vi "指令集合.vi"() -> ()   [LabVIEW 2016]
uses:
  Global variable.vi
  <vilib>/addons/_office/excel.llb/Excel Get Data ([str]).vi
  <vilib>/regexp/Match Regular Expression.xnode
  <vilib>/Utility/NIReport.llb/NI_report.lvclass
  <vilib>/Utility/NIReport.llb/Excel/NI_Excel.lvclass
  <vilib>/addons/_office/NI_ReportGenerationToolkit.lvlib
panel:
  in  "Tab Control":T1(tab)
  in  "get_error":bool
  in  "ooc or b update":enum16{"b update", "ooc update", "ooc&b update"}(ring)
  in  "打快门":bool
  in  "数据源":T2(ring)
  in  "byPathSel":enum16{"0", "1"}(ring)=enum."1"
  in  "KBC":bool=TRUE
  in  "AGC":bool=TRUE
  in  "HBC":bool=TRUE
  in  "VBC":bool=TRUE
  in  "TNR":bool=TRUE
  in  "SNR":bool=TRUE
  in  "GAMMA":bool=TRUE
  in  "像素取反":bool
  in  "去锅盖":bool=TRUE
  in  "对焦使能":bool
  in  "Blind_rp_en":bool
  in  "VISA resource name":refnum<visa-resource-name>
  in  "COM":bool
  in  "快门片使能":bool=TRUE
  in  "快门片开合":bool=TRUE
  in  "get_vtemp":bool
  out "return":i32
  out "vtemp":u16
  in  "命令集合":string(combo)
  in  "指令窗口":string
  out "指令触发":bool
  out "error out":errorcluster
  in  "new_dead_pix":u8[](array[numeric])
  out "String_out":string
  in  "String_in":string
  in  "Enum":enum16{"number", "hex", "string"}(ring)
  in  "数值":u8
  in  "长度":u16
  in  "加载到data_in":bool
  in  "data数组清空":bool
  out "data_out":u8[](array[numeric])
  in  "data_in":u8[](array[numeric])
  in  "standard_get":bool
  in  "standard_send":bool
  in  "std_byCmdType":string
  in  "std_bySubCmd":string
  in  "std_byPara":string
  in  "std_byAddr_h":string
  in  "std_wAddr":string
  in  "std_wLength":string
  in  "cmd_std_header_t":T3
  out "standard_send_return":i32
  out "standard_get_return":i32
  in  "Boolean":bool
  out "读取字符串（16进制）":string
  in  "写入字符串（16进制）":string
  in  "写入长度":string
  in  "写入地址（16进制）":string
  in  "读取地址（16进制）":string
  in  "读取长度":string
  in  "寄存器写入":bool
  in  "寄存器读取":bool
  in  "long_dwLen":string
  in  "long_dwAddr2":string
  in  "long_dwAddr1":string
  in  "long_wPara":string
  in  "long_bySubCmd":string
  in  "long_byCmd":string
  in  "long_get":bool
  in  "long_send":bool
  in  "vd_cmd_long_header_t":T4
  out "long_send_return":i32
  out "long_data out":u8[](array[numeric])
  out "long_get_return":i32
  in  "osd_get":bool
  in  "osd_send":bool
  out "osd_get_return":i32
  out "osd_data out":u8[](array[numeric])
  out "osd_send_return":i32
  in  "osd_byCmd":string
  in  "osd_bySubcmd":string
  in  "osd_byIndex":string
  in  "osd_byPara":string
  in  "osd_data_in":u8[](array[numeric])
  out "快门开合":i32
  out "快门使能":i32
  out "Blind_rp_en R":i32
  out "像素取反 return":i32
  out "读取寄存器":i32
  out "写入寄存器":i32
  out "GAMMA return":i32
  out "AGC return":i32
  out "SNR return":i32
  out "TNR return":i32
  out "VBC return":i32
  out "HBC return":i32
  out "去锅盖 return":i32
  out "KBC return":i32
  out "对焦使能 2":i32
  out "Y16start":i32
  out "Y16stop":i32
  out "oocBupdate":i32
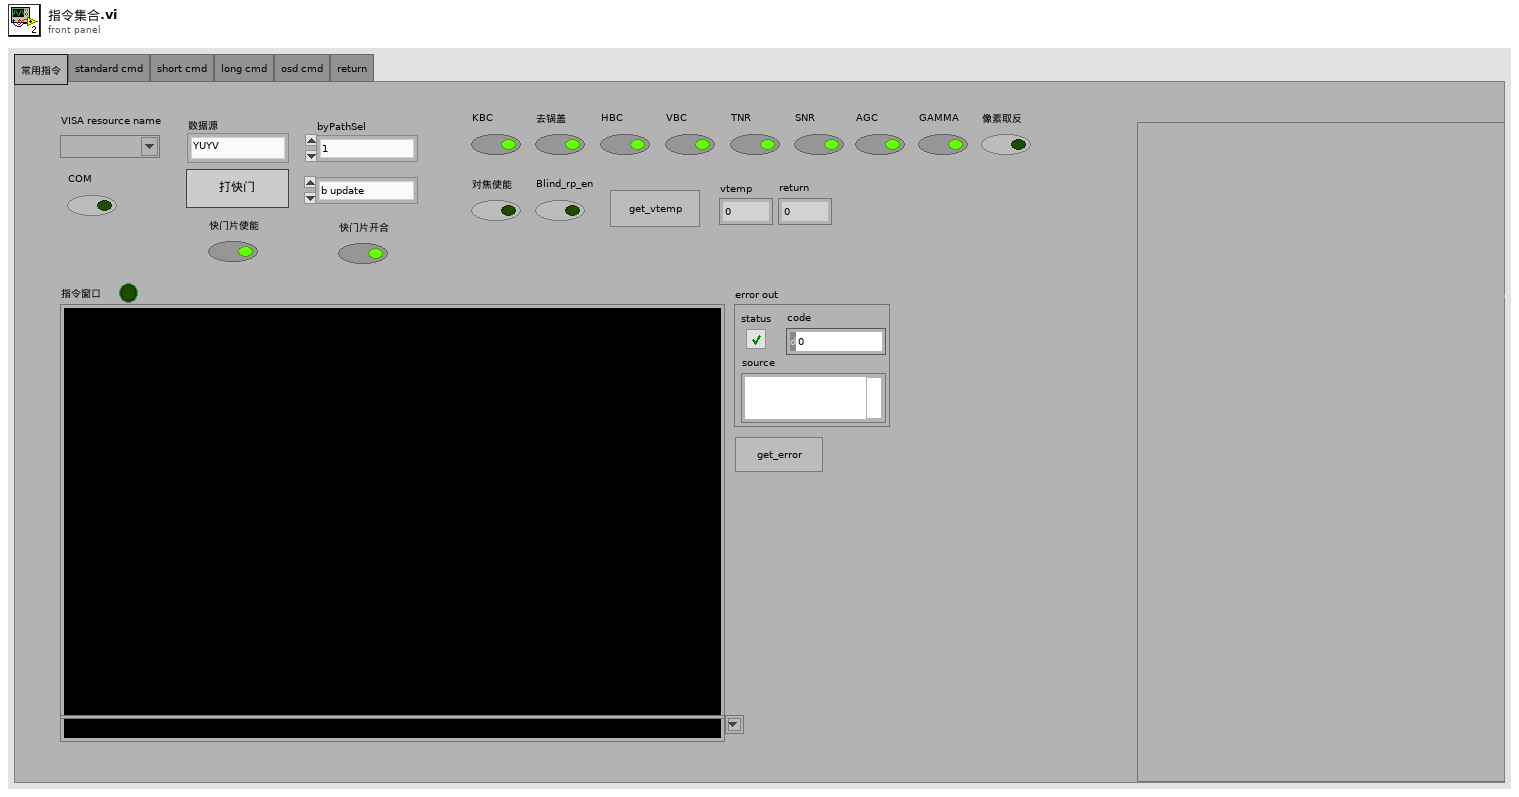
[diagram p1: front panel]
types:
  T1 = enum32{"常用指令", "standard cmd", "short cmd", "long cmd", "osd cmd", "return"}
  T2 = enum16{"YUYV", "TEMPERATURE", "IR", "KBC", "HBC_DPC", "VBC", "TNR", "SNR", "AGC", "DDE", "GAMMA", "MIRROR"}
  T3 = cluster{"byCmdType":u8, "bySubCmd":u8, "byPara":u8, "byAddr_h":u8, "byAddr_l":u8, "byAddr_ll":u8, "byLen_h":u8, "byLen_l":u8}
  T4 = cluster{"byCmd":u8, "bySubCmd":u8, "byParam_h":u8, "byParam_l":u8, "byAddr1_hh":u8, "byAddr1_h":u8, "byAddr1_l":u8, "byAddr1_ll":u8, "byAddr2_hh":u8, "byAddr2_h":u8, "byAddr2_l":u8, "byAddr2_ll":u8, "byLen_hh":u8, "byLen_h":u8, "byLen_l":u8, "byLen_ll":u8}
  T5 = enum16{"Standard Report", "HTML", "Word", "Excel"}
  T6 = enum16{"maximized", "minimized", "normal", "no change"}
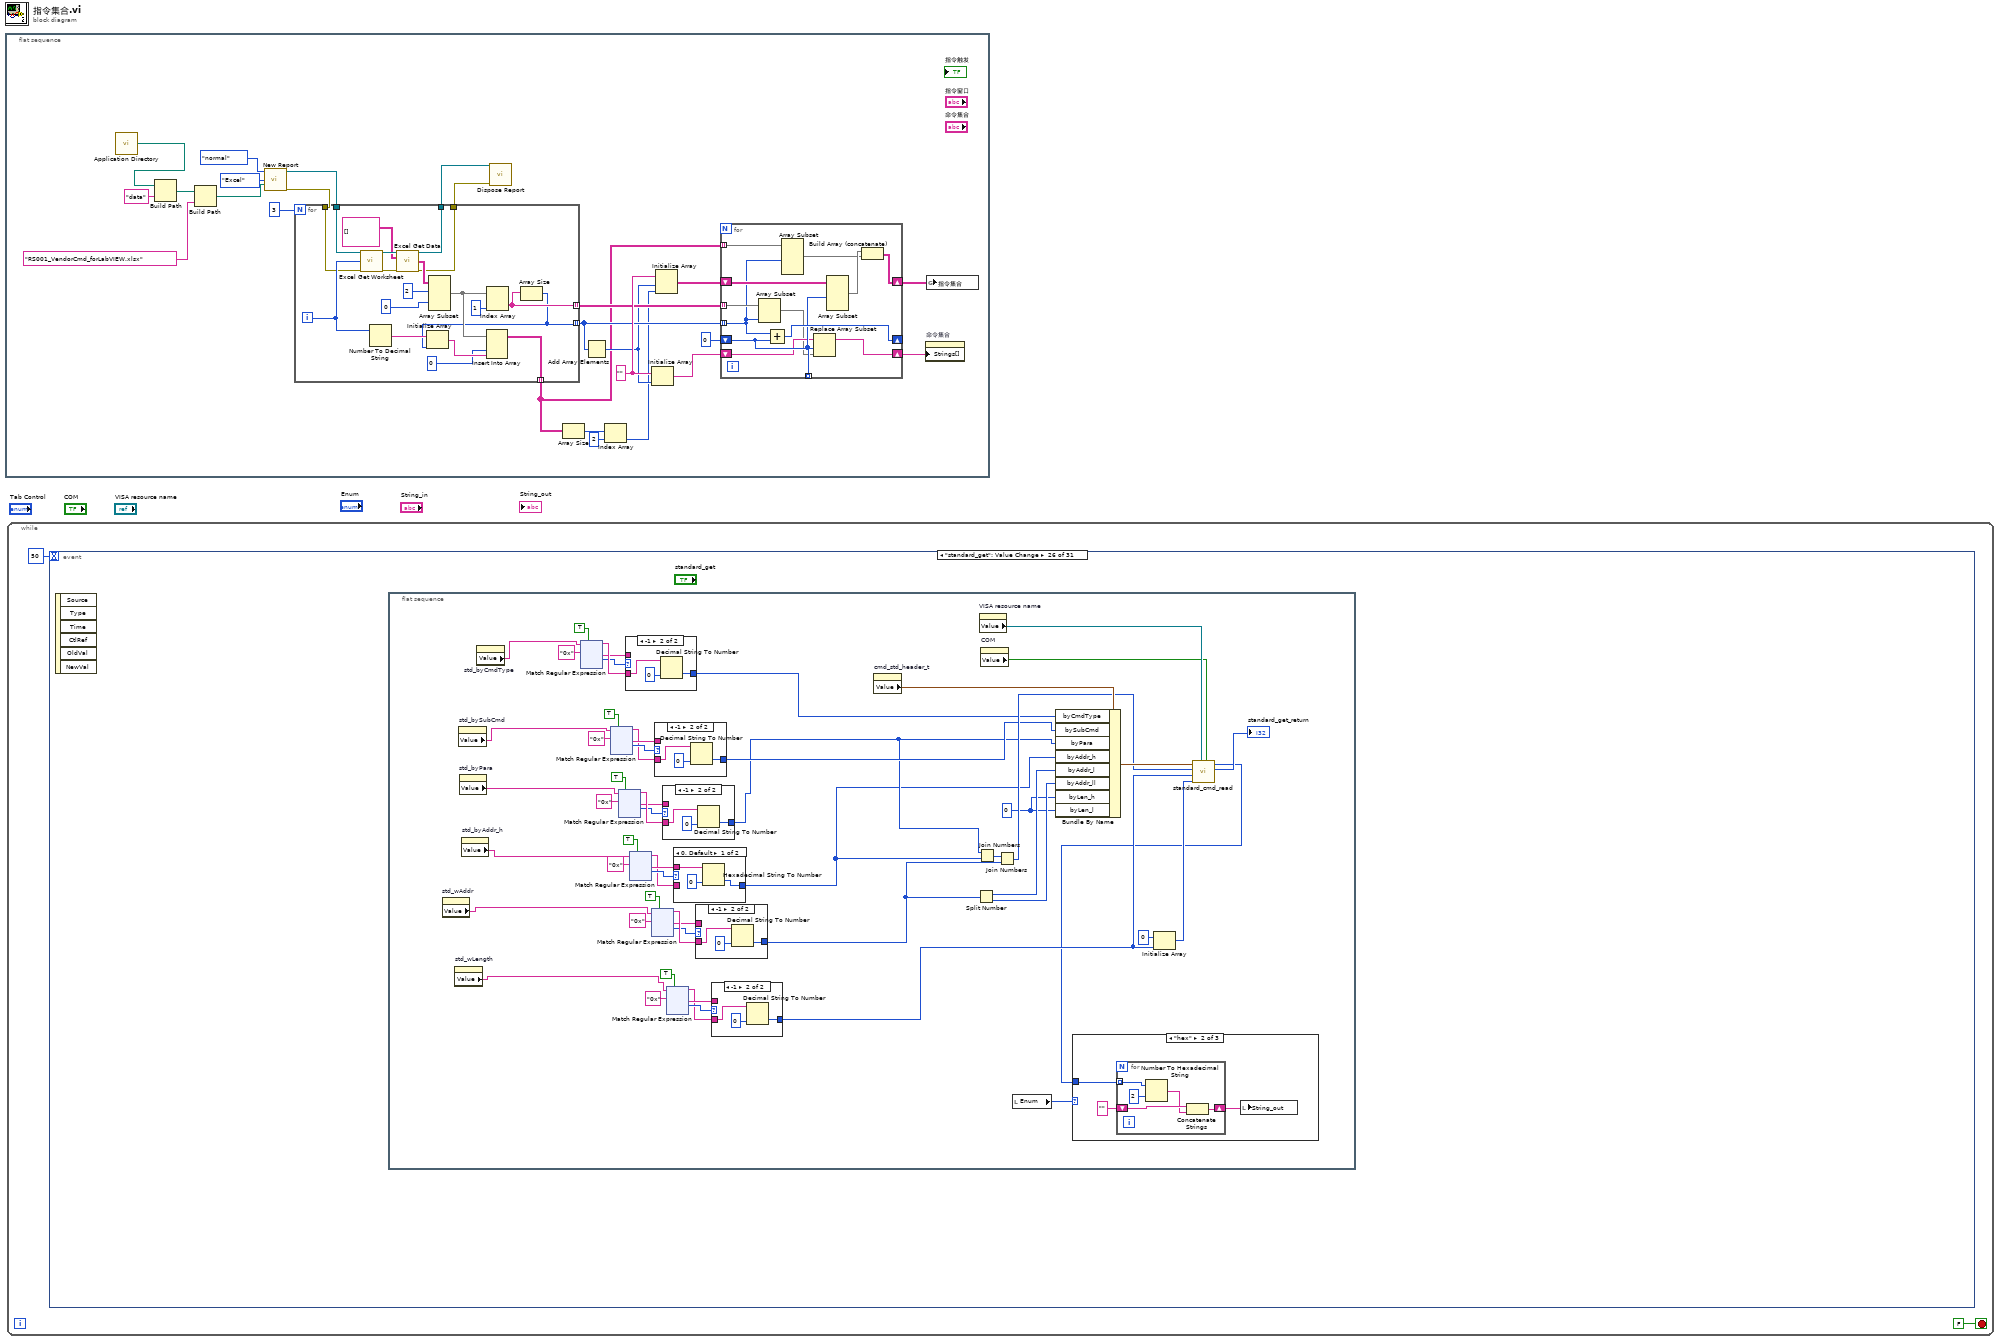
[diagram p0: block diagram]
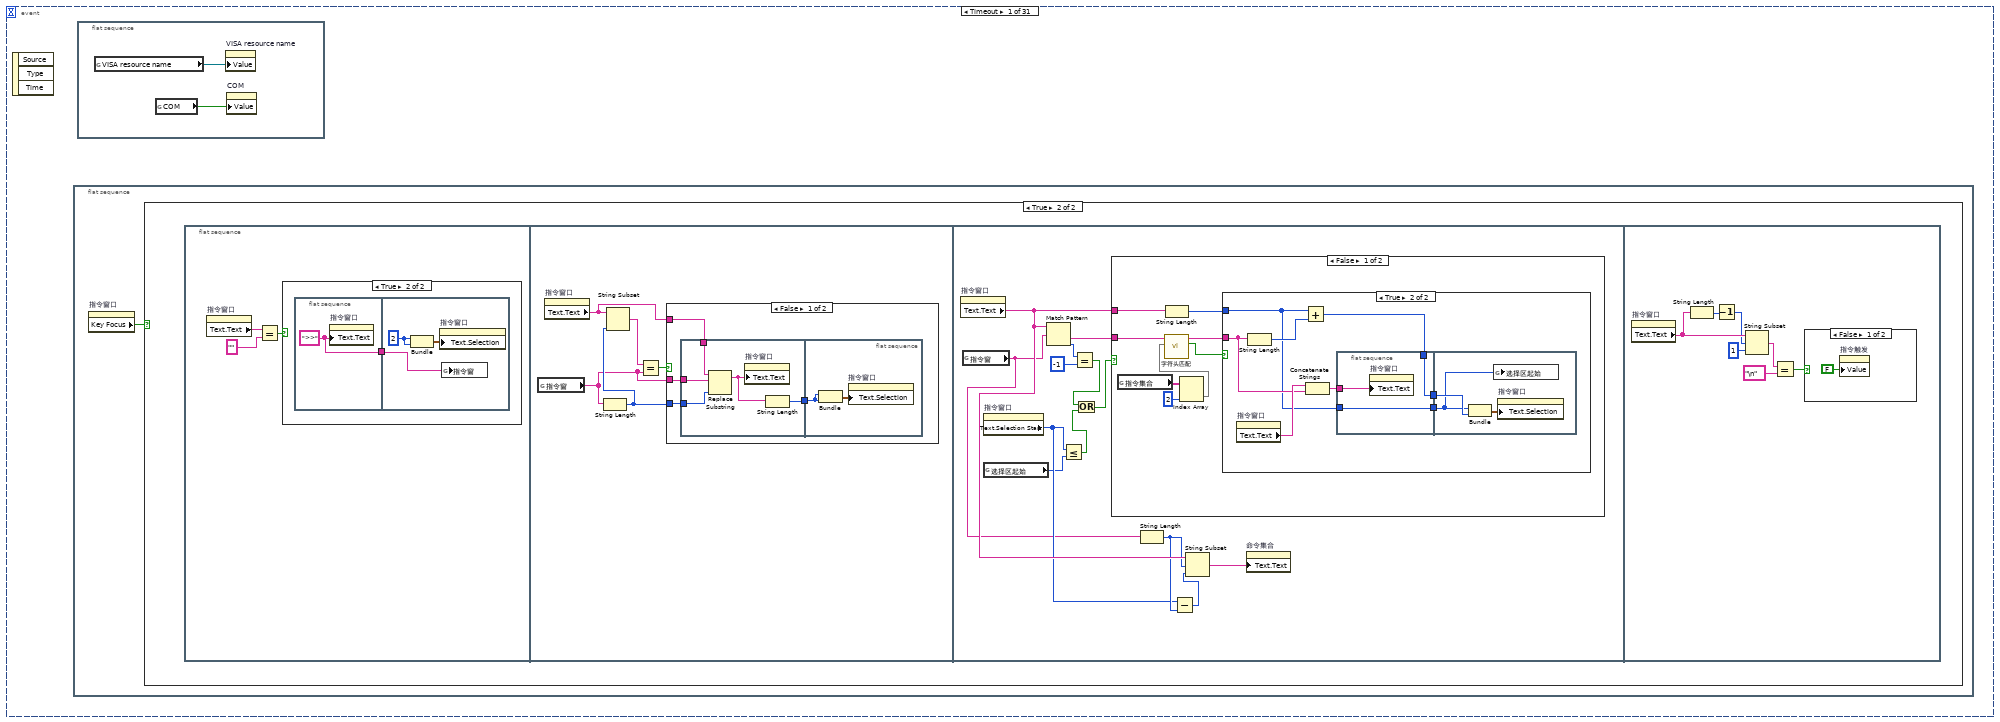
[diagram p2: hidden frame]
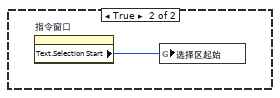
[diagram p7: hidden frame]
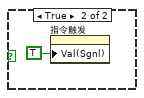
[diagram p8: hidden frame]
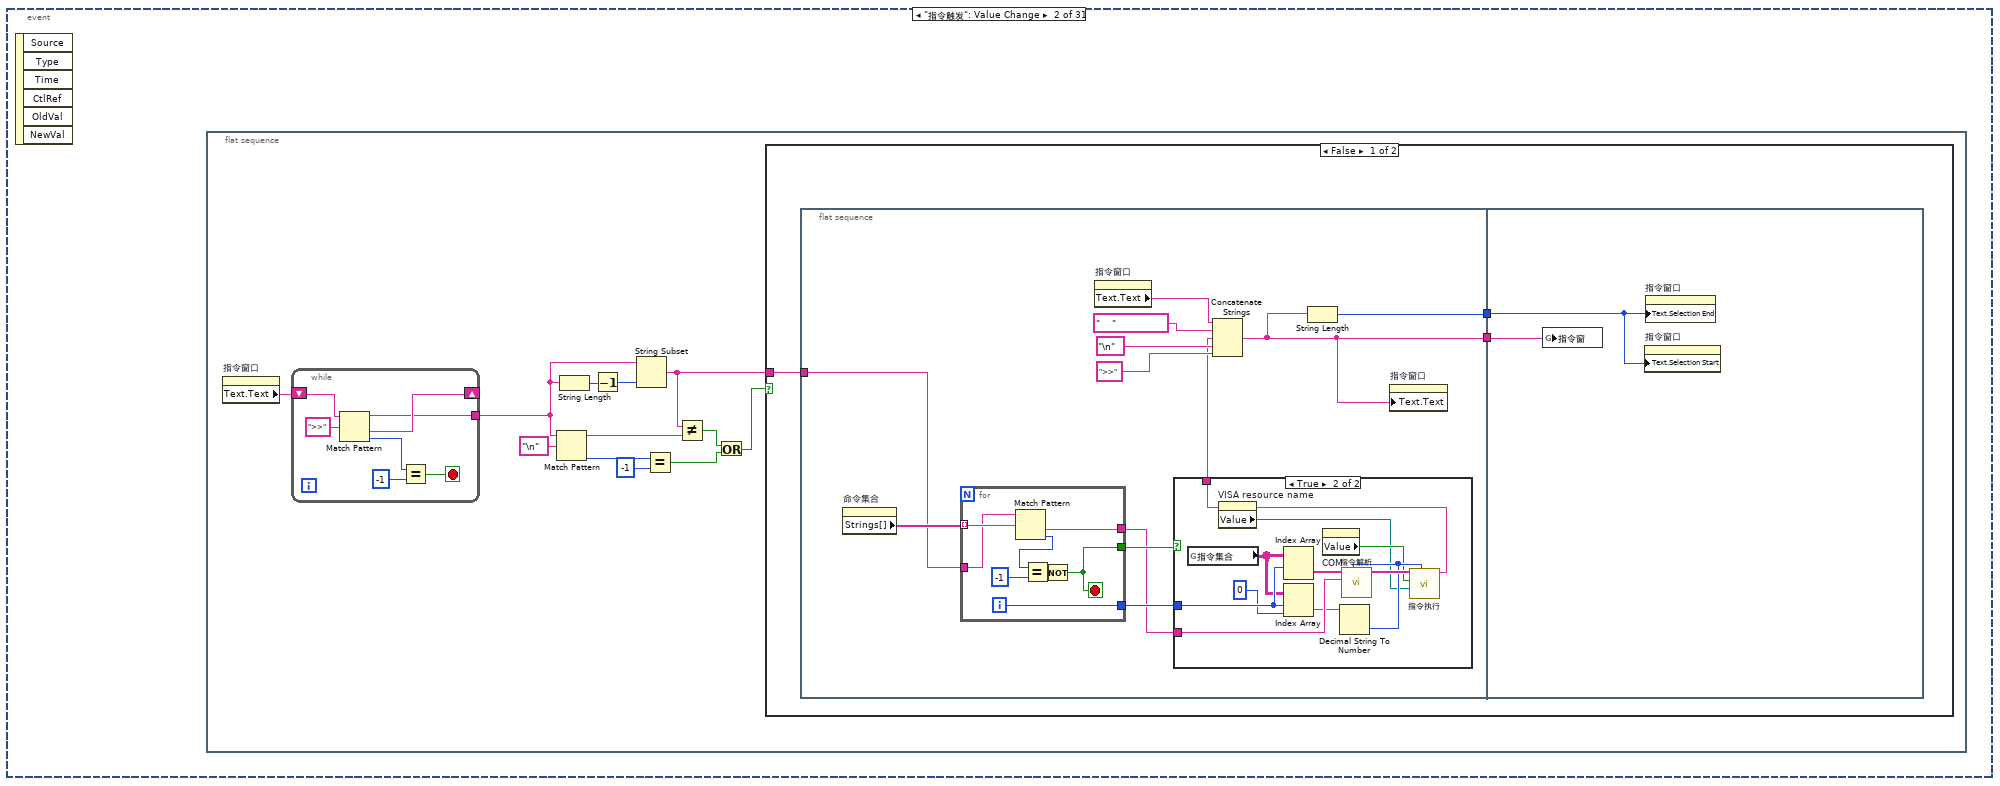
[diagram p9: hidden frame]
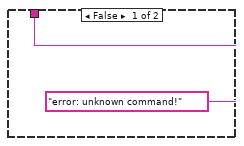
[diagram p10: hidden frame]
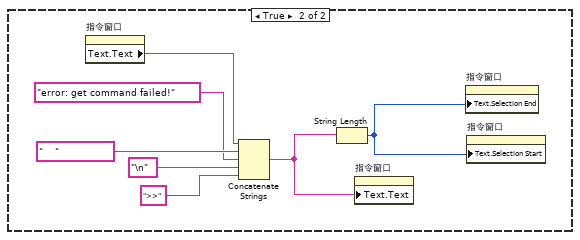
[diagram p11: hidden frame]
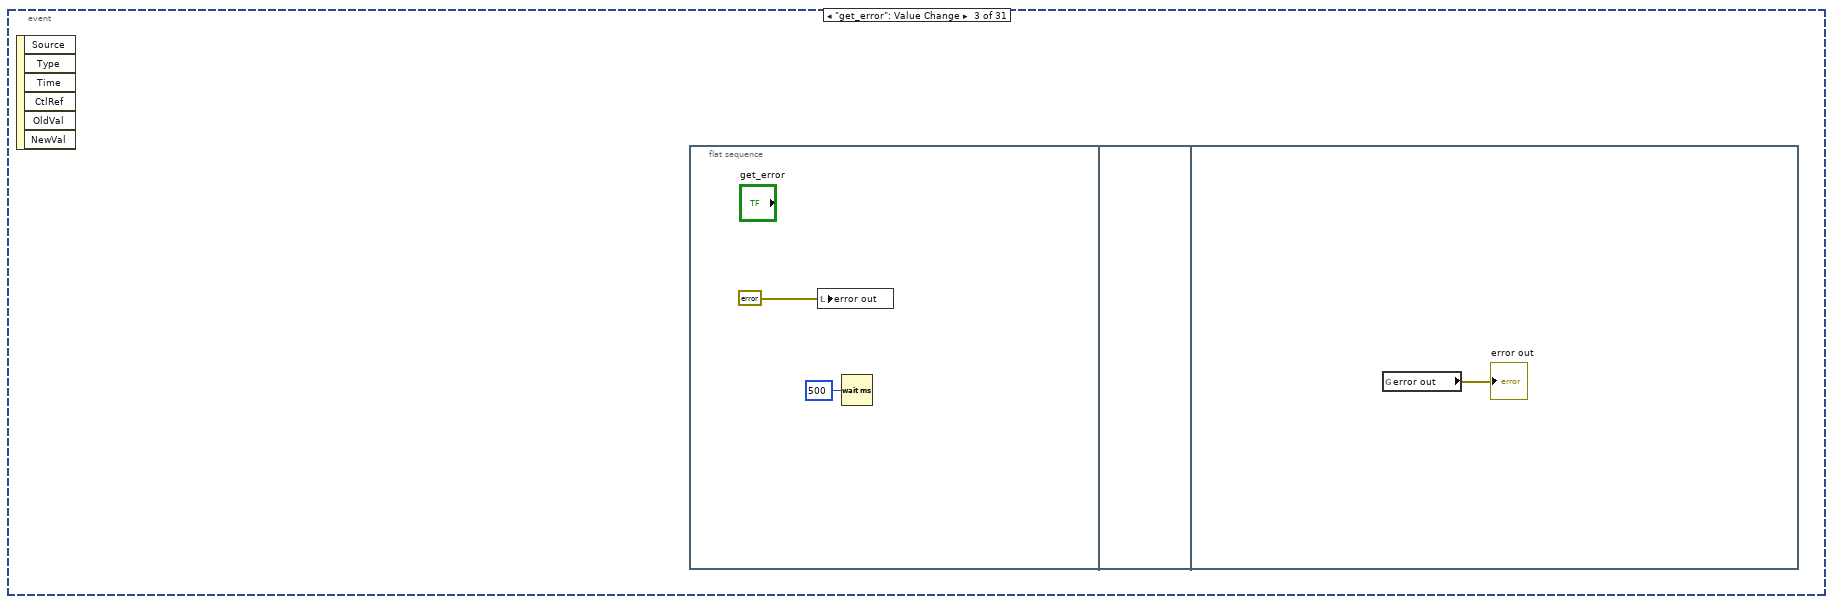
[diagram p12: hidden frame]
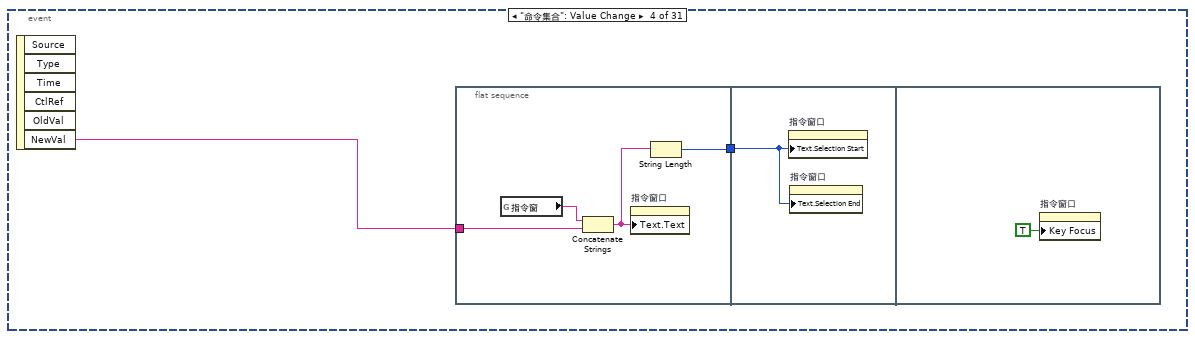
[diagram p13: hidden frame]
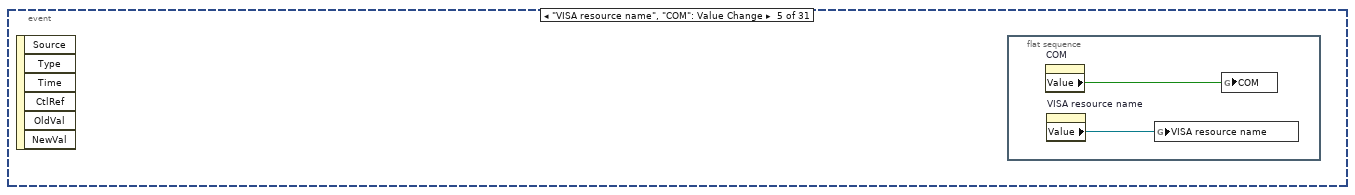
[diagram p14: hidden frame]
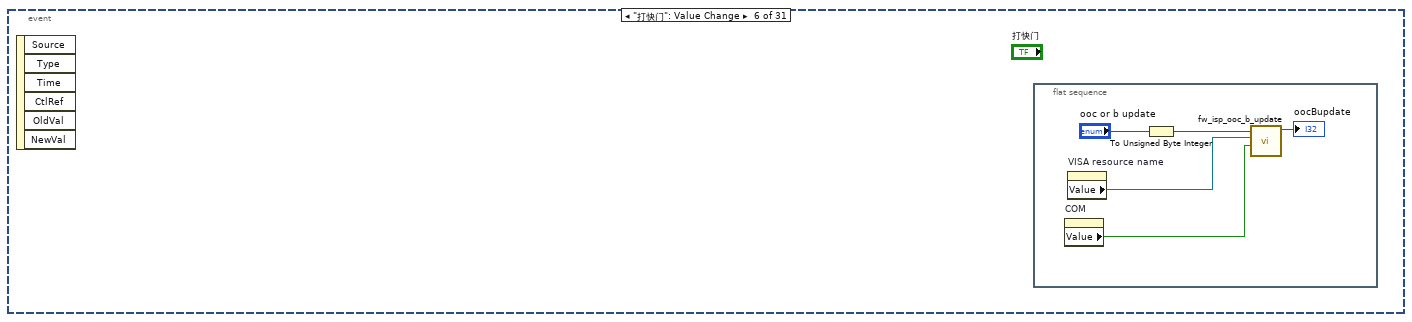
[diagram p15: hidden frame]
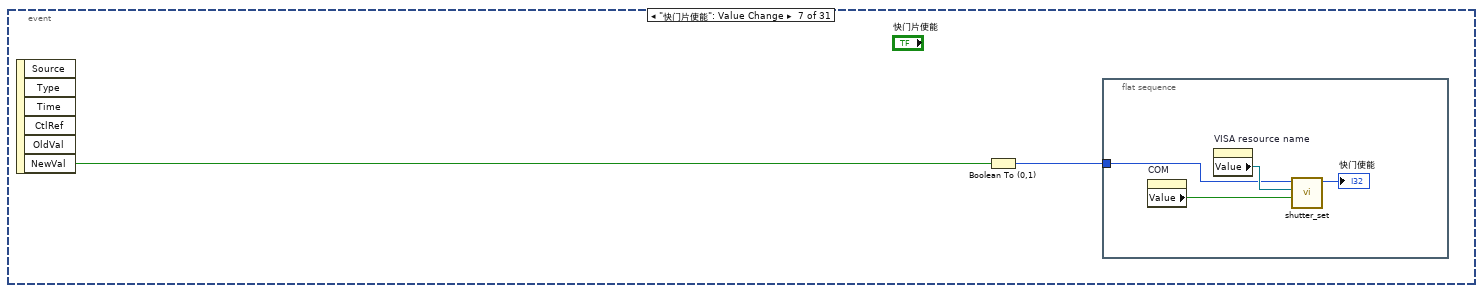
[diagram p16: hidden frame]
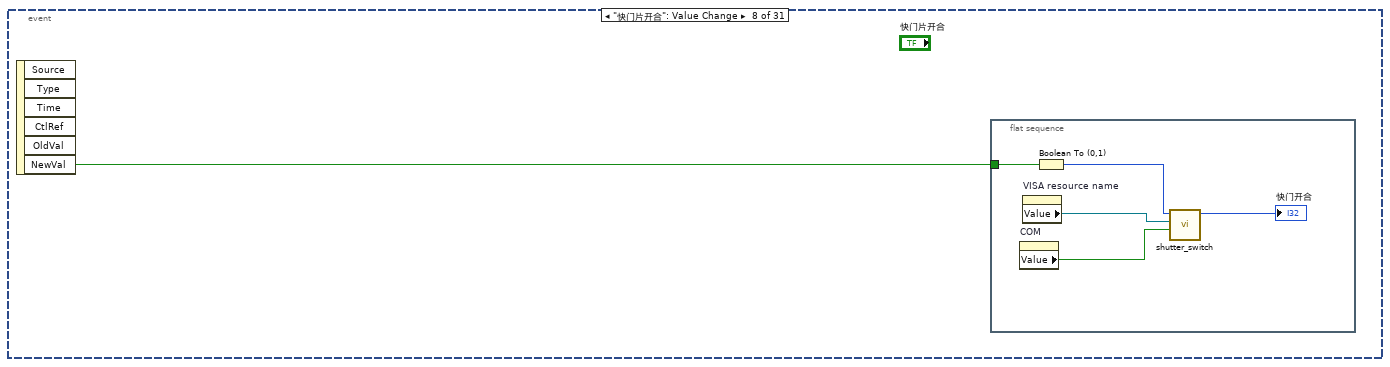
[diagram p17: hidden frame]
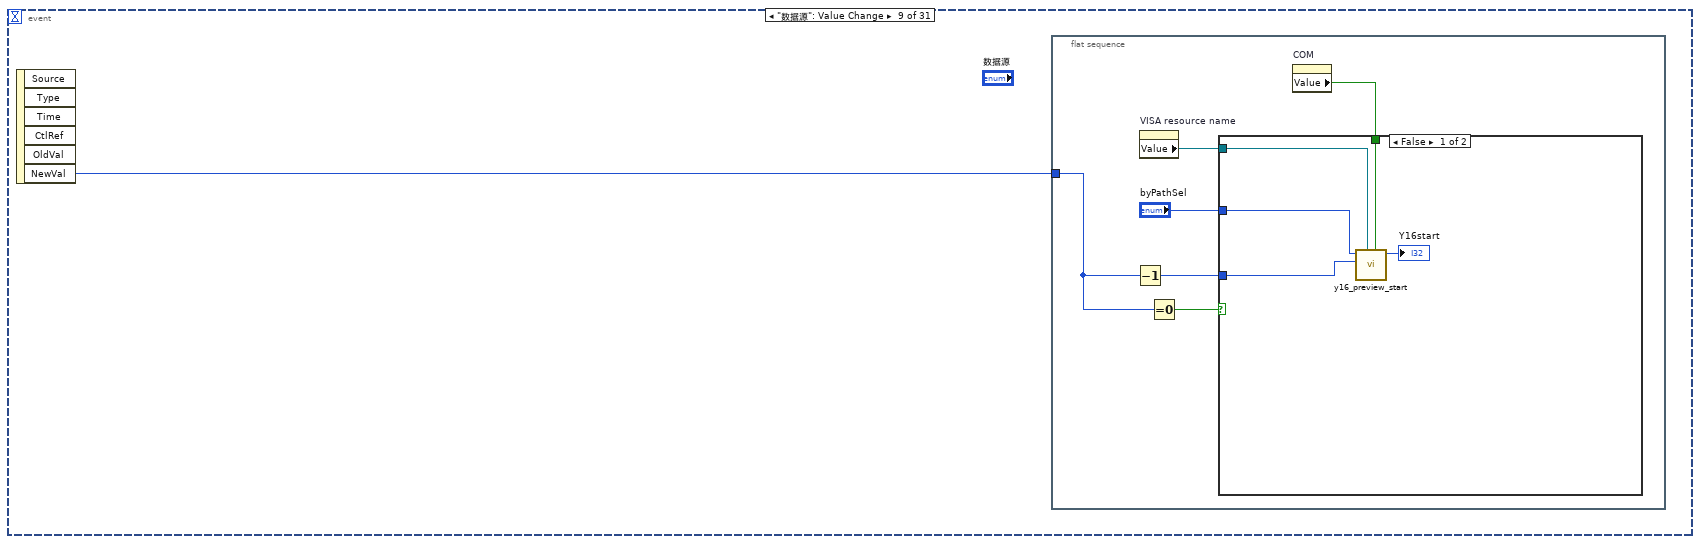
[diagram p18: hidden frame]
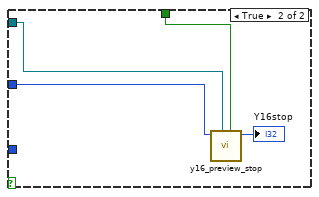
[diagram p19: hidden frame]
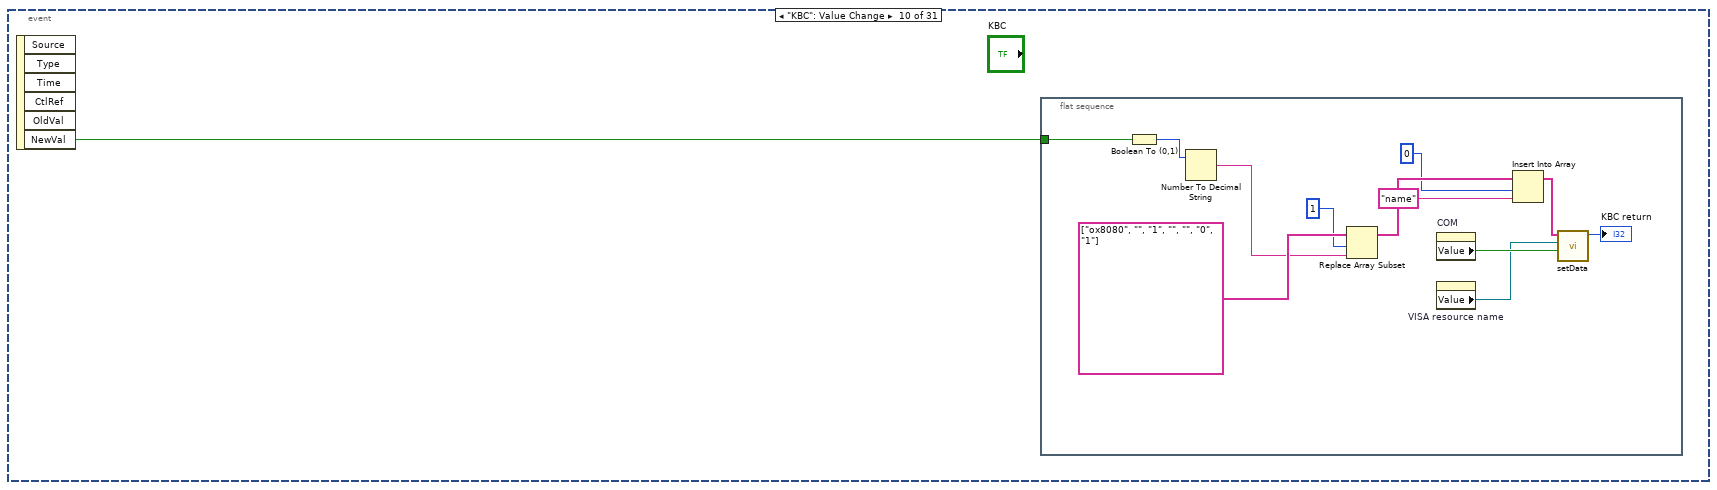
[diagram p20: hidden frame]
diagram:
  n1 = flat-sequence {
    frame #0 {
      w24 = ""
      n2 = call <vilib>:"Application Directory.vi"() -> ("Application Directory"=w2:path)
      n3 = Build Path(base path=w2, name or relative path="data") -> (appended path=w3:path)
      n4 = Build Path(base path=w3, name or relative path="RS001_VendorCmd_forLabVIEW.xlsx" ("名称或相对路径")) -> (appended path=w5:path)
      n5 = call <vilib>:"New Report.vi"("window state (normal)"=T6."normal", "report type"=T5."Excel", "template (empty)"=w5) -> ("report out"=w10:refnum<class "NI_report.lvclass">, "error out"=w9:errorcluster)  [unwired: 11 in]
      n6 = for {
        N: 3 -> [_]
        tunnel: [w49] -> w21 mode=indexing
        tunnel: [w43] -> w12 mode=indexing
        tunnel: [w42] -> w20 mode=indexing
        tunnel: w10 -> [w41]
        tunnel: w9 -> [w40]
        tunnel: [w39] -> w8
        tunnel: [w38] -> w7
        i -> [w48]
        n7 = call <vilib>:"Excel Get Worksheet.vi"("report in"=w41, "worksheet index (0)"=w48, "error in (no error)"=w40) -> ("report out"=w54:refnum<class "NI_report.lvclass">, "error out"=w55:errorcluster)  [unwired: 11 in]
        n8 = Number To Decimal String(number=w48) -> (decimal integer string=w47:string)  [unwired: 1 in]
        n9 = call-poly <vilib>:"Excel Get Data.vi"("report in"=w54, "data type"=string[][] [], "error in (no error)"=w55) -> ("report out"=w39:refnum<class "NI_report.lvclass">, "data"=w56:string[][], "error out"=w38:errorcluster)  [unwired: 10 in]
        n10 = Array Subset(array=w56, index (row)=2 ("索引"), index (col)=0 ("索引")) -> (w46:string[][])  [unwired: 2 in]
        n11 = Index Array(array=w46, index (col)=1 ("禁用的索引 (列)")) -> (element=w49:string[])  [unwired: 1 in]
        n12 = Array Size(array=w49) -> (size(s)=w42:i32)
        n13 = Initialize Array(w47, w42) -> (w45:string[])
        n14 = Insert Into Array(array=w46, index (col)=0 ("禁用的索引 (列)"), new element=w45) -> (w43:string[][])  [unwired: 1 in]
      }
      n15 = call-dynamic "Dispose Report.vi"("report in"=w8, "error in (no error)"=w7) -> ()  [unwired: 13 in, 1 out]
      n16 = Array Size(array=w12) -> (size(s)=w23:i32[])
      n17 = Add Array Elements(numeric array=w20) -> (sum=w14:i32)
      n18 = Index Array(array=w23, index=2 ("索引")) -> (element=w13:i32)
      n19 = Initialize Array(w24, w14) -> (w19:string[])
      n20 = Initialize Array(w24, w14, w13) -> (w18:string[][])
      n21 = for {
        tunnel: w21 -> [w37] mode=indexing
        tunnel: w20 -> [w32] mode=indexing
        shift-right: [w36] -> w16
        shift-left: w19 -> [w27]
        shift-right: [w29] -> w15
        shift-left: w18 -> [w34]
        shift-right: [w35] -> _
        shift-left: 0 -> [w28]
        tunnel: w12 -> [w33] mode=indexing
        tunnel: [w28] -> _ mode=indexing
        n22 = Array Subset(array=w37, length=w32) -> (w26:string[])  [unwired: 1 in]
        n23 = Add(x=w32, y=w28) -> (x+y=w35:i32)
        n24 = Array Subset(array=w33, length (row)=w32) -> (w30:string[][])  [unwired: 3 in]
        n25 = Replace Array Subset(array=w27, new element=w26, index=w28) -> (w36:string[])
        n26 = Array Subset(array=w34, length (row)=w28) -> (w31:string[][])  [unwired: 3 in]
        n27 = Build Array (concatenate)(w31, w30) -> (w29:string[][])
      }
      n28 = property on="命令集合" class="CmbBox"("Strings[]"=w16) -> ()  [unwired: 2 in, 2 out]
      n29 = global write "Global variable.vi" "指令集合"(w15) -> ()
    }
  }
  n30 = while {
    stop <- FALSE stop-if-true
    n31 = event shown="[25] \"standard_get\": Value Change" {
      selector: _ -> [_ _ _ _ _ _ _ _ _ _ _ _ _ _ _ _ _ _ _ _ _ _ _ _ _ _ _ _ _ _ _]
      dyn-events: _ -> [_ _ _ _ _ _ _ _ _ _ _ _ _ _ _ _ _ _ _ _ _ _ _ _ _ _ _ _ _ _ _]
      timeout: 50 -> [_ _ _ _ _ _ _ _ _ _ _ _ _ _ _ _ _ _ _ _ _ _ _ _ _ _ _ _ _ _ _]
      event Timeout {
        n32 = event-data() -> ()  [unwired: 1 in, 3 out]
        n33 = flat-sequence {
          frame #0 {
            n34 = property on="指令窗口" class="Str"() -> ("Key Focus"=w59:bool)  [unwired: 2 in, 2 out]
            n35 = case shown="True" w59 {
              frame False {
              }
              frame True {
                n36 = flat-sequence {
                  frame #0 {
                    n37 = property on="指令窗口" class="Str"() -> ("Text.Text"=w60:string)  [unwired: 2 in, 2 out]
                    n38 = Equal?(x=w60, y="") -> (x = y?=w62:bool)
                    n39 = case shown="True" w62 {
                      frame False {
                      }
                      frame True {
                        n40 = flat-sequence {
                          tunnel: [w64] -> w63
                          tunnel: w63 -> [w65]
                          frame #0 {
                            w64 = ">>" ("文本.文本")
                            n41 = property on="指令窗口" class="Str"("Text.Text"=w64) -> ()  [unwired: 2 in, 2 out]
                          }
                          frame #1 {
                            w66 = u32 2
                            n42 = Bundle(w66, w66) -> (w67:cluster{u32, u32})  [unwired: 1 in]
                            n43 = property on="指令窗口" class="Str"("Text.Selection"=w67) -> ()  [unwired: 2 in, 2 out]
                            n44 = global write "Global variable.vi" "指令窗"(w65) -> ()
                          }
                        }
                      }
                    }
                  }
                  frame #1 {
                    n45 = global read "Global variable.vi" "指令窗"() -> (w68:string)
                    n46 = property on="指令窗口" class="Str"() -> ("Text.Text"=w69:string)  [unwired: 2 in, 2 out]
                    n47 = String Length(string=w68) -> (length=w70:i32)
                    n48 = String Subset(string=w69, length (rest)=w70) -> (substring=w71:string)  [unwired: 1 in]
                    n49 = Equal?(x=w71, y=w68) -> (x = y?=w72:bool)
                    n50 = case shown="False" w72 {
                      tunnel: w68 -> [w76 _]
                      tunnel: w69 -> [w75 _]
                      tunnel: w70 -> [w74 _]
                      frame False {
                        n51 = flat-sequence {
                          tunnel: w76 -> [w81]
                          tunnel: w75 -> [w80]
                          tunnel: w74 -> [w79]
                          tunnel: [w77] -> w73
                          tunnel: w73 -> [w82]
                          frame #0 {
                            n52 = Replace Substring(2:w79, 4:w81, 5:w80) -> (1:w78:string)  [unwired: 1 in, 1 out]
                            n53 = property on="指令窗口" class="Str"("Text.Text"=w78) -> ()  [unwired: 2 in, 2 out]
                            n54 = String Length(string=w78) -> (length=w77:i32)
                          }
                          frame #1 {
                            n55 = Bundle(w82, w82) -> (w83:cluster{i32, i32})  [unwired: 1 in]
                            n56 = property on="指令窗口" class="Str"("Text.Selection"=w83) -> ()  [unwired: 2 in, 2 out]
                          }
                        }
                      }
                      frame True {
                      }
                    }
                  }
                  frame #2 {
                    n57 = property on="指令窗口" class="Str"() -> ("Text.Text"=w90:string)  [unwired: 2 in, 2 out]
                    n58 = global read "Global variable.vi" "指令窗"() -> (w85:string)
                    n59 = property on="指令窗口" class="Str"() -> ("Text.Selection Start"=w86:u32)  [unwired: 2 in, 2 out]
                    n60 = global read "Global variable.vi" "选择区起始"() -> (w84:u32)
                    n61 = Match Pattern(string=w90, regular expression=w85) -> (after substring=w94:string, offset past match=w96:i32)  [unwired: 1 in, 2 out]
                    n62 = Less Or Equal?(x=w86, y=w84) -> (x <= y?=w91:bool)
                    n63 = Equal?(x=w96, y=-1) -> (x = y?=w92:bool)
                    n64 = Or(x=w92, y=w91) -> (x .or. y?=w93:bool)
                    n65 = case shown="False" w93 {
                      tunnel: w94 -> [w104 _]
                      tunnel: w90 -> [w99 _]
                      frame False {
                        n66 = global read "Global variable.vi" "指令集合"() -> (w97:string[][])
                        n67 = String Length(string=w99) -> (length=w98:i32)
                        n68 = Index Array(array=w97, index (col)=2 ("禁用的索引 (列)")) -> (element=w102:string[])  [unwired: 1 in]
                        n69 = call "字符头匹配.vi"("匹配字符数组"=w102, "字符头"=w104) -> ("匹配结果"=w101:bool, "匹配之后"=w100:string)  [unwired: 8 in]
                        n70 = case shown="True" w101 {
                          tunnel: w100 -> [_ w111]
                          tunnel: w98 -> [_ w107]
                          frame False {
                          }
                          frame True {
                            n71 = property on="指令窗口" class="Str"() -> ("Text.Text"=w112:string)  [unwired: 2 in, 2 out]
                            n72 = String Length(string=w111) -> (length=w110:i32)
                            n73 = Add(x=w107, y=w110) -> (x+y=w108:i32)
                            n74 = Concatenate Strings(w112, w111) -> (w109:string)
                            n75 = flat-sequence {
                              tunnel: w109 -> [w113]
                              tunnel: w108 -> [w114]
                              tunnel: w107 -> [w115]
                              tunnel: [w115] -> w106
                              tunnel: [w114] -> w105
                              tunnel: w106 -> [w116]
                              tunnel: w105 -> [w117]
                              frame #0 {
                                n76 = property on="指令窗口" class="Str"("Text.Text"=w113) -> ()  [unwired: 2 in, 2 out]
                              }
                              frame #1 {
                                n77 = Bundle(w116, w117) -> (w118:cluster{i32, i32})  [unwired: 1 in]
                                n78 = global write "Global variable.vi" "选择区起始"(w116) -> ()
                                n79 = property on="指令窗口" class="Str"("Text.Selection"=w118) -> ()  [unwired: 2 in, 2 out]
                              }
                            }
                          }
                        }
                      }
                      frame True {
                        n80 = property on="指令窗口" class="Str"() -> ("Text.Selection Start"=w119:u32)  [unwired: 2 in, 2 out]
                        n81 = global write "Global variable.vi" "选择区起始"(w119) -> ()
                      }
                    }
                    n82 = String Length(string=w85) -> (length=w89:i32)
                    n83 = Subtract(x=w86, y=w89) -> (x-y=w88:u32)
                    n84 = String Subset(string=w90, offset (0)=w89, length (rest)=w88) -> (substring=w87:string)
                    n85 = property on="命令集合" class="CmbBox"("Text.Text"=w87) -> ()  [unwired: 2 in, 2 out]
                  }
                  frame #3 {
                    n86 = property on="指令窗口" class="Str"() -> ("Text.Text"=w126:string)  [unwired: 2 in, 2 out]
                    n87 = String Length(string=w126) -> (length=w125:i32)
                    n88 = Decrement(x=w125) -> (x-1=w124:i32)
                    n89 = String Subset(string=w126, offset (0)=w124, length (rest)=1 ("长度（剩余）")) -> (substring=w122:string)
                    n90 = Equal?(x=w122, y="\n") -> (x = y?=w120:bool)
                    n91 = case shown="False" w120 {
                      frame False {
                        n92 = property on="指令触发" class="Bool (strict)"("Value"=FALSE ("指令触发")) -> ()  [unwired: 2 in, 2 out]
                      }
                      frame True {
                        n93 = property on="指令触发" class="Bool (strict)"("Val(Sgnl)"=TRUE ("值(信号)")) -> ()  [unwired: 2 in, 2 out]
                      }
                    }
                  }
                }
              }
            }
          }
        }
        n94 = flat-sequence {
          frame #0 {
            n95 = global read "Global variable.vi" "VISA resource name"() -> (w130:refnum<visa-resource-name>)
            n96 = global read "Global variable.vi" "COM"() -> (w129:bool)
            n97 = property on="VISA resource name" class="VISAName"("Value"=w130) -> ()  [unwired: 2 in, 2 out]
            n98 = property on="COM" class="Bool (strict)"("Value"=w129) -> ()  [unwired: 2 in, 2 out]
          }
        }
      }
      event "指令触发": Value Change {
        n99 = event-data() -> ()  [unwired: 1 in, 6 out]
        n100 = flat-sequence {
          frame #0 {
            n101 = property on="指令窗口" class="Str"() -> ("Text.Text"=w131:string)  [unwired: 2 in, 2 out]
            n102 = while {
              shift-right: [w191] -> _
              shift-left: w131 -> [w193]
              tunnel: [w187] -> w141
              stop <- w188 stop-if-true
              n103 = Match Pattern(string=w193, regular expression=">>" ("正则表达式")) -> (before substring=w187:string, after substring=w191:string, offset past match=w190:i32)  [unwired: 1 in, 1 out]
              n104 = Equal?(x=w190, y=-1) -> (x = y?=w188:bool)
            }
            n105 = Match Pattern(string=w141, regular expression="\n" ("正则表达式")) -> (before substring=w138:string, offset past match=w137:i32)  [unwired: 1 in, 2 out]
            n106 = String Length(string=w141) -> (length=w140:i32)
            n107 = Decrement(x=w140) -> (x-1=w139:i32)
            n108 = String Subset(string=w141, length (rest)=w139) -> (substring=w132:string)  [unwired: 1 in]
            n109 = Equal?(x=w137, y=-1) -> (x = y?=w134:bool)
            n110 = Not Equal?(x=w132, y=w138) -> (x != y?=w135:bool)
            n111 = Or(x=w135, y=w134) -> (x .or. y?=w133:bool)
            n112 = case shown="False" w133 {
              tunnel: w132 -> [w145 _]
              frame False {
                n113 = flat-sequence {
                  tunnel: w145 -> [w147]
                  tunnel: [w149] -> w144
                  tunnel: [w148] -> w143
                  tunnel: w144 -> [w179]
                  tunnel: w143 -> [w178]
                  frame #0 {
                    n114 = property on="命令集合" class="CmbBox"() -> ("Strings[]"=w154:string[])  [unwired: 2 in, 2 out]
                    n115 = for {
                      tunnel: w154 -> [w175] mode=indexing
                      tunnel: w147 -> [w174]
                      tunnel: [w173] -> w153
                      tunnel: [w176] -> w151
                      tunnel: [w170] -> w146
                      i -> [w176]
                      stop <- w173 stop-if-true
                      n116 = Match Pattern(string=w174, regular expression=w175) -> (after substring=w170:string, offset past match=w172:i32)  [unwired: 1 in, 2 out]
                      n117 = Equal?(x=w172, y=-1) -> (x = y?=w177:bool)
                      n118 = Not(x=w177) -> (.not. x?=w173:bool)
                    }
                    n119 = property on="指令窗口" class="Str"() -> ("Text.Text"=w150:string)  [unwired: 2 in, 2 out]
                    n120 = case shown="True" w153 {
                      tunnel: ["error: unknown command!" ("字符串") w162] -> w152
                      tunnel: w151 -> [_ w167]
                      tunnel: w146 -> [_ w168]
                      frame False {
                      }
                      frame True {
                        n121 = global read "Global variable.vi" "指令集合"() -> (w161:string[][])
                        n122 = property on="VISA resource name" class="VISAName"() -> ("Value"=w159:refnum<visa-resource-name>)  [unwired: 2 in, 2 out]
                        n123 = Index Array(array=w161, index (row)=w167) -> (element=w169:string[])  [unwired: 1 in]
                        n124 = Index Array(array=w161, index (row)=w167, index (col)=0 ("索引 (列)")) -> (element=w165:string)
                        n125 = property on="COM" class="Bool (strict)"() -> ("Value"=w160:bool)  [unwired: 2 in, 2 out]
                        n126 = Decimal String To Number(string=w165) -> (number=w163:i32)  [unwired: 2 in, 1 out]
                        n127 = call "指令解析.vi"("指令类型"=w163, "参数字符串"=w168, "指令数组输入"=w169) -> ("指令输出"=w164:string[])  [unwired: 8 in]
                        n128 = call "指令执行.vi"("指令类型"=w163, "VISA name"=w159, "COM"=w160, "参数数组输入"=w164) -> ("结果输出"=w162:string)  [unwired: 7 in]
                      }
                    }
                    n129 = Concatenate Strings(w150, "    " ("字符串"), w152, "\n" ("字符串"), ">>" ("字符串")) -> (w148:string)
                    n130 = String Length(string=w148) -> (length=w149:i32)
                    n131 = property on="指令窗口" class="Str"("Text.Text"=w148) -> ()  [unwired: 2 in, 2 out]
                  }
                  frame #1 {
                    n132 = global write "Global variable.vi" "指令窗"(w178) -> ()
                    n133 = property on="指令窗口" class="Str"("Text.Selection Start"=w179) -> ()  [unwired: 2 in, 2 out]
                    n134 = property on="指令窗口" class="Str"("Text.Selection End"=w179) -> ()  [unwired: 2 in, 2 out]
                  }
                }
              }
              frame True {
                n135 = property on="指令窗口" class="Str"() -> ("Text.Text"=w182:string)  [unwired: 2 in, 2 out]
                n136 = Concatenate Strings(w182, "    " ("字符串"), "error: get command failed!" ("字符串"), "\n" ("字符串"), ">>" ("字符串")) -> (w181:string)
                n137 = String Length(string=w181) -> (length=w180:i32)
                n138 = property on="指令窗口" class="Str"("Text.Text"=w181) -> ()  [unwired: 2 in, 2 out]
                n139 = property on="指令窗口" class="Str"("Text.Selection End"=w180) -> ()  [unwired: 2 in, 2 out]
                n140 = property on="指令窗口" class="Str"("Text.Selection Start"=w180) -> ()  [unwired: 2 in, 2 out]
              }
            }
          }
        }
      }
      event "get_error": Value Change {
        n141 = event-data() -> ()  [unwired: 1 in, 6 out]
        n142 = flat-sequence {
          frame #0 {
            n143 = local write "error out"(errorcluster {"status"=FALSE, "code"=0, "source"=""} ("error out")) -> ()
            n144 = Wait (ms)(milliseconds to wait=u32 500) -> ()  [unwired: 1 out]
          }
          frame #1 {
          }
          frame #2 {
            n145 = global read "Global variable.vi" "error out"() -> (→"error out":errorcluster)
          }
        }
      }
      event "命令集合": Value Change {
        n146 = event-data() -> ("NewVal"=w197:string)  [unwired: 1 in, 5 out]
        n147 = flat-sequence {
          tunnel: w197 -> [w201]
          tunnel: [w199] -> w198
          tunnel: w198 -> [w203]
          frame #0 {
            n148 = global read "Global variable.vi" "指令窗"() -> (w202:string)
            n149 = Concatenate Strings(w202, w201) -> (w200:string)
            n150 = property on="指令窗口" class="Str"("Text.Text"=w200) -> ()  [unwired: 2 in, 2 out]
            n151 = String Length(string=w200) -> (length=w199:i32)
          }
          frame #1 {
            n152 = property on="指令窗口" class="Str"("Text.Selection Start"=w203) -> ()  [unwired: 2 in, 2 out]
            n153 = property on="指令窗口" class="Str"("Text.Selection End"=w203) -> ()  [unwired: 2 in, 2 out]
          }
          frame #2 {
            n154 = property on="指令窗口" class="Str"("Key Focus"=TRUE ("键选中")) -> ()  [unwired: 2 in, 2 out]
          }
        }
      }
      event "VISA resource name", "COM": Value Change {
        n155 = event-data() -> ()  [unwired: 1 in, 6 out]
        n156 = flat-sequence {
          frame #0 {
            n157 = property on="COM" class="Bool (strict)"() -> ("Value"=w206:bool)  [unwired: 2 in, 2 out]
            n158 = property on="VISA resource name" class="VISAName"() -> ("Value"=w205:refnum<visa-resource-name>)  [unwired: 2 in, 2 out]
            n159 = global write "Global variable.vi" "VISA resource name"(w205) -> ()
            n160 = global write "Global variable.vi" "COM"(w206) -> ()
          }
        }
      }
      event "打快门": Value Change {
        n161 = event-data() -> ()  [unwired: 1 in, 6 out]
        n162 = flat-sequence {
          frame #0 {
            n163 = property on="COM" class="Bool (strict)"() -> ("Value"=w207:bool)  [unwired: 2 in, 2 out]
            n164 = property on="VISA resource name" class="VISAName"() -> ("Value"=w208:refnum<visa-resource-name>)  [unwired: 2 in, 2 out]
            n165 = To Unsigned Byte Integer(number="ooc or b update") -> (unsigned 8bit integer=w209:u8)
            n166 = call "fw_isp_ooc_b_update.vi"("COM"=w207, "VISA name"=w208, "eUpdateType(0 or 1 or 2)"=w209) -> ("return"=→"oocBupdate":i32)  [unwired: 8 in]
          }
        }
      }
      event "快门片使能": Value Change {
        n167 = event-data() -> ("NewVal"=w213:bool)  [unwired: 1 in, 5 out]
        n168 = Boolean To (0,1)(Boolean=w213) -> (0, 1=w212:i16)
        n169 = flat-sequence {
          tunnel: w212 -> [w216]
          frame #0 {
            n170 = property on="COM" class="Bool (strict)"() -> ("Value"=w215:bool)  [unwired: 2 in, 2 out]
            n171 = property on="VISA resource name" class="VISAName"() -> ("Value"=w217:refnum<visa-resource-name>)  [unwired: 2 in, 2 out]
            n172 = call "shutter_set.vi"("COM"=w215, "VISA name"=w217, "eSwitchType 0 or 1"=w216) -> ("return"=→"快门使能":i32)  [unwired: 8 in]
          }
        }
      }
      event "快门片开合": Value Change {
        n173 = event-data() -> ("NewVal"=w218:bool)  [unwired: 1 in, 5 out]
        n174 = flat-sequence {
          tunnel: w218 -> [w221]
          frame #0 {
            n175 = property on="COM" class="Bool (strict)"() -> ("Value"=w223:bool)  [unwired: 2 in, 2 out]
            n176 = property on="VISA resource name" class="VISAName"() -> ("Value"=w222:refnum<visa-resource-name>)  [unwired: 2 in, 2 out]
            n177 = Boolean To (0,1)(Boolean=w221) -> (0, 1=w220:i16)
            n178 = call "shutter_switch.vi"("COM"=w223, "VISA name"=w222, "eSwitchType 0 or 1"=w220) -> ("return"=→"快门开合":i32)  [unwired: 8 in]
          }
        }
      }
      event "数据源": Value Change {
        n179 = event-data() -> ("NewVal"=w224:T2)  [unwired: 1 in, 5 out]
        n180 = flat-sequence {
          tunnel: w224 -> [w229]
          frame #0 {
            n181 = Decrement(x=w229) -> (x-1=w227:T2)
            n182 = property on="VISA resource name" class="VISAName"() -> ("Value"=w225:refnum<visa-resource-name>)  [unwired: 2 in, 2 out]
            n183 = Equal To 0?(x=w229) -> (x = 0?=w230:bool)
            n184 = property on="COM" class="Bool (strict)"() -> ("Value"=w226:bool)  [unwired: 2 in, 2 out]
            n185 = case shown="False" w230 {
              tunnel: w227 -> [w235 _]
              tunnel: "byPathSel" -> [w233 w238]
              tunnel: w226 -> [w232 w236]
              tunnel: w225 -> [w231 w237]
              frame False {
                n186 = call "y16_preview_start.vi"("COM"=w232, "VISA name"=w231, "byISPStreamSrcSel"=w235, "byPath"=w233) -> ("return"=→"Y16start":i32)  [unwired: 7 in]
              }
              frame True {
                n187 = call "y16_preview_stop.vi"("COM"=w236, "VISA name"=w237, "byPath"=w238) -> ("return"=→"Y16stop":i32)  [unwired: 8 in]
              }
            }
          }
        }
      }
      event "KBC": Value Change {
        n188 = event-data() -> ("NewVal"=w240:bool)  [unwired: 1 in, 5 out]
        n189 = flat-sequence {
          tunnel: w240 -> [w252]
          frame #0 {
            n190 = Boolean To (0,1)(Boolean=w252) -> (0, 1=w251:i16)
            n191 = Number To Decimal String(number=w251) -> (decimal integer string=w248:string)  [unwired: 1 in]
            n192 = Replace Array Subset(array=string[] ["ox8080", "", "1", "", "", "0", "1"], new element=w248, index=1) -> (w246:string[])
            n193 = property on="COM" class="Bool (strict)"() -> ("Value"=w242:bool)  [unwired: 2 in, 2 out]
            n194 = property on="VISA resource name" class="VISAName"() -> ("Value"=w241:refnum<visa-resource-name>)  [unwired: 2 in, 2 out]
            n195 = Insert Into Array(array=w246, index=0, new element="name" ("new element/subarray")) -> (w243:string[])
            n196 = call "setData.vi"("COM"=w242, "VISA name"=w241, "Array"=w243) -> ("return"=→"KBC return":i32)  [unwired: 8 in]
          }
        }
      }
      event "去锅盖": Value Change {
        n197 = event-data() -> ("NewVal"=w253:bool)  [unwired: 1 in, 5 out]
        n198 = flat-sequence {
          tunnel: w253 -> [w261]
          frame #0 {
            n199 = Boolean To (0,1)(Boolean=w261) -> (0, 1=w265:i16)
            n200 = Number To Decimal String(number=w265) -> (decimal integer string=w262:string)  [unwired: 1 in]
            n201 = Replace Array Subset(array=string[] ["ox8740", "", "1", "", "", "3", "1"], new element=w262, index=1) -> (w257:string[])
            n202 = property on="COM" class="Bool (strict)"() -> ("Value"=w255:bool)  [unwired: 2 in, 2 out]
            n203 = property on="VISA resource name" class="VISAName"() -> ("Value"=w254:refnum<visa-resource-name>)  [unwired: 2 in, 2 out]
            n204 = Insert Into Array(array=w257, index=0, new element="name" ("new element/subarray")) -> (w256:string[])
            n205 = call "setData.vi"("COM"=w255, "VISA name"=w254, "Array"=w256) -> ("return"=→"去锅盖 return":i32)  [unwired: 8 in]
          }
        }
      }
      event "HBC": Value Change {
        n206 = event-data() -> ("NewVal"=w266:bool)  [unwired: 1 in, 5 out]
        n207 = flat-sequence {
          tunnel: w266 -> [w274]
          frame #0 {
            n208 = Boolean To (0,1)(Boolean=w274) -> (0, 1=w278:i16)
            n209 = Number To Decimal String(number=w278) -> (decimal integer string=w275:string)  [unwired: 1 in]
            n210 = Replace Array Subset(array=string[] ["ox8200", "", "1", "", "", "0", "1"], new element=w275, index=1) -> (w270:string[])
            n211 = property on="VISA resource name" class="VISAName"() -> ("Value"=w267:refnum<visa-resource-name>)  [unwired: 2 in, 2 out]
            n212 = property on="COM" class="Bool (strict)"() -> ("Value"=w268:bool)  [unwired: 2 in, 2 out]
            n213 = Insert Into Array(array=w270, index=0, new element="name" ("new element/subarray")) -> (w269:string[])
            n214 = call "setData.vi"("COM"=w268, "VISA name"=w267, "Array"=w269) -> ("return"=→"HBC return":i32)  [unwired: 8 in]
          }
        }
      }
      event "VBC": Value Change {
        n215 = event-data() -> ("NewVal"=w279:bool)  [unwired: 1 in, 5 out]
        n216 = flat-sequence {
          tunnel: w279 -> [w287]
          frame #0 {
            n217 = Boolean To (0,1)(Boolean=w287) -> (0, 1=w291:i16)
            n218 = Number To Decimal String(number=w291) -> (decimal integer string=w288:string)  [unwired: 1 in]
            n219 = Replace Array Subset(array=string[] ["ox8300", "", "1", "", "", "0", "1"], new element=w288, index=1) -> (w283:string[])
            n220 = property on="COM" class="Bool (strict)"() -> ("Value"=w281:bool)  [unwired: 2 in, 2 out]
            n221 = property on="VISA resource name" class="VISAName"() -> ("Value"=w280:refnum<visa-resource-name>)  [unwired: 2 in, 2 out]
            n222 = Insert Into Array(array=w283, index=0, new element="name" ("new element/subarray")) -> (w282:string[])
            n223 = call "setData.vi"("COM"=w281, "VISA name"=w280, "Array"=w282) -> ("return"=→"VBC return":i32)  [unwired: 8 in]
          }
        }
      }
      event "TNR": Value Change {
        n224 = event-data() -> ("NewVal"=w292:bool)  [unwired: 1 in, 5 out]
        n225 = flat-sequence {
          tunnel: w292 -> [w300]
          frame #0 {
            n226 = Boolean To (0,1)(Boolean=w300) -> (0, 1=w304:i16)
            n227 = Number To Decimal String(number=w304) -> (decimal integer string=w301:string)  [unwired: 1 in]
            n228 = Replace Array Subset(array=string[] ["ox8400", "", "1", "", "", "7", "1"], new element=w301, index=1) -> (w296:string[])
            n229 = property on="VISA resource name" class="VISAName"() -> ("Value"=w293:refnum<visa-resource-name>)  [unwired: 2 in, 2 out]
            n230 = property on="COM" class="Bool (strict)"() -> ("Value"=w294:bool)  [unwired: 2 in, 2 out]
            n231 = Insert Into Array(array=w296, index=0, new element="name" ("new element/subarray")) -> (w295:string[])
            n232 = call "setData.vi"("COM"=w294, "VISA name"=w293, "Array"=w295) -> ("return"=→"TNR return":i32)  [unwired: 8 in]
          }
        }
      }
      event "SNR": Value Change {
        n233 = event-data() -> ("NewVal"=w305:bool)  [unwired: 1 in, 5 out]
        n234 = flat-sequence {
          tunnel: w305 -> [w313]
          frame #0 {
            n235 = Boolean To (0,1)(Boolean=w313) -> (0, 1=w317:i16)
            n236 = Number To Decimal String(number=w317) -> (decimal integer string=w314:string)  [unwired: 1 in]
            n237 = Replace Array Subset(array=string[] ["ox8500", "", "1", "", "", "0", "1"], new element=w314, index=1) -> (w309:string[])
            n238 = property on="COM" class="Bool (strict)"() -> ("Value"=w307:bool)  [unwired: 2 in, 2 out]
            n239 = property on="VISA resource name" class="VISAName"() -> ("Value"=w306:refnum<visa-resource-name>)  [unwired: 2 in, 2 out]
            n240 = Insert Into Array(array=w309, index=0, new element="name" ("new element/subarray")) -> (w308:string[])
            n241 = call "setData.vi"("COM"=w307, "VISA name"=w306, "Array"=w308) -> ("return"=→"SNR return":i32)  [unwired: 8 in]
          }
        }
      }
      event "AGC": Value Change {
        n242 = event-data() -> ("NewVal"=w318:bool)  [unwired: 1 in, 5 out]
        n243 = flat-sequence {
          tunnel: w318 -> [w327]
          frame #0 {
            n244 = Not(x=w327) -> (.not. x?=w321:bool)
            n245 = Boolean To (0,1)(Boolean=w321) -> (0, 1=w331:i16)
            n246 = Number To Decimal String(number=w331) -> (decimal integer string=w328:string)  [unwired: 1 in]
            n247 = Replace Array Subset(array=string[] ["ox85A4", "", "1", "", "", "2", "1"], new element=w328, index=1) -> (w323:string[])
            n248 = property on="VISA resource name" class="VISAName"() -> ("Value"=w319:refnum<visa-resource-name>)  [unwired: 2 in, 2 out]
            n249 = property on="COM" class="Bool (strict)"() -> ("Value"=w320:bool)  [unwired: 2 in, 2 out]
            n250 = Insert Into Array(array=w323, index=0, new element="name" ("new element/subarray")) -> (w322:string[])
            n251 = call "setData.vi"("COM"=w320, "VISA name"=w319, "Array"=w322) -> ("return"=→"AGC return":i32)  [unwired: 8 in]
          }
        }
      }
      event "GAMMA": Value Change {
        n252 = event-data() -> ("NewVal"=w332:bool)  [unwired: 1 in, 5 out]
        n253 = flat-sequence {
          tunnel: w332 -> [w340]
          frame #0 {
            n254 = Boolean To (0,1)(Boolean=w340) -> (0, 1=w344:i16)
            n255 = Number To Decimal String(number=w344) -> (decimal integer string=w341:string)  [unwired: 1 in]
            n256 = Replace Array Subset(array=string[] ["ox8700", "", "1", "", "", "0", "1"], new element=w341, index=1) -> (w336:string[])
            n257 = property on="VISA resource name" class="VISAName"() -> ("Value"=w333:refnum<visa-resource-name>)  [unwired: 2 in, 2 out]
            n258 = Insert Into Array(array=w336, index=0, new element="name" ("new element/subarray")) -> (w335:string[])
            n259 = property on="COM" class="Bool (strict)"() -> ("Value"=w334:bool)  [unwired: 2 in, 2 out]
            n260 = call "setData.vi"("COM"=w334, "VISA name"=w333, "Array"=w335) -> ("return"=→"GAMMA return":i32)  [unwired: 8 in]
          }
        }
      }
      event "像素取反": Value Change {
        n261 = event-data() -> ("NewVal"=w345:bool)  [unwired: 1 in, 5 out]
        n262 = flat-sequence {
          tunnel: w345 -> [w353]
          frame #0 {
            n263 = Boolean To (0,1)(Boolean=w353) -> (0, 1=w357:i16)
            n264 = Number To Decimal String(number=w357) -> (decimal integer string=w356:string)  [unwired: 1 in]
            n265 = Replace Array Subset(array=string[] ["ox8700", "", "1", "", "", "4", "1"], new element=w356, index=1) -> (w349:string[])
            n266 = property on="VISA resource name" class="VISAName"() -> ("Value"=w346:refnum<visa-resource-name>)  [unwired: 2 in, 2 out]
            n267 = property on="COM" class="Bool (strict)"() -> ("Value"=w347:bool)  [unwired: 2 in, 2 out]
            n268 = Insert Into Array(array=w349, index=0, new element="name" ("new element/subarray")) -> (w348:string[])
            n269 = call "setData.vi"("COM"=w347, "VISA name"=w346, "Array"=w348) -> ("return"=→"像素取反 return":i32)  [unwired: 8 in]
          }
        }
      }
      event "对焦使能": Value Change {
        n270 = event-data() -> ("NewVal"=w358:bool)  [unwired: 1 in, 5 out]
        n271 = flat-sequence {
          tunnel: w358 -> [w362]
          frame #0 {
            n272 = Boolean To (0,1)(Boolean=w362) -> (0, 1=w370:i16)
            n273 = Number To Decimal String(number=w370) -> (decimal integer string=w369:string)  [unwired: 1 in]
            n274 = Replace Array Subset(array=string[] ["ox8500", "", "1", "", "", "1", "1"], new element=w369, index=1) -> (w368:string[])
            n275 = property on="VISA resource name" class="VISAName"() -> ("Value"=w359:refnum<visa-resource-name>)  [unwired: 2 in, 2 out]
            n276 = property on="COM" class="Bool (strict)"() -> ("Value"=w360:bool)  [unwired: 2 in, 2 out]
            n277 = Insert Into Array(array=w368, index=0, new element="name" ("new element/subarray")) -> (w367:string[])
            n278 = call "setData.vi"("COM"=w360, "VISA name"=w359, "Array"=w367) -> ("return"=→"对焦使能 2":i32)  [unwired: 8 in]
          }
        }
      }
      event "Blind_rp_en": Value Change {
        n279 = event-data() -> ("NewVal"=w371:bool)  [unwired: 1 in, 5 out]
        n280 = flat-sequence {
          tunnel: w371 -> [w375]
          frame #0 {
            n281 = Boolean To (0,1)(Boolean=w375) -> (0, 1=w383:i16)
            n282 = Number To Decimal String(number=w383) -> (decimal integer string=w382:string)  [unwired: 1 in]
            n283 = Replace Array Subset(array=string[] ["ox8500", "", "1", "", "", "2", "1"], new element=w382, index=1) -> (w381:string[])
            n284 = property on="VISA resource name" class="VISAName"() -> ("Value"=w372:refnum<visa-resource-name>)  [unwired: 2 in, 2 out]
            n285 = property on="COM" class="Bool (strict)"() -> ("Value"=w373:bool)  [unwired: 2 in, 2 out]
            n286 = Insert Into Array(array=w381, index=0, new element="name" ("new element/subarray")) -> (w380:string[])
            n287 = call "setData.vi"("COM"=w373, "VISA name"=w372, "Array"=w380) -> ("return"=→"Blind_rp_en R":i32)  [unwired: 8 in]
          }
        }
      }
      event "寄存器写入": Value Change {
        n288 = event-data() -> ()  [unwired: 1 in, 6 out]
        n289 = flat-sequence {
          frame #0 {
            n290 = xnode "Match Regular Expression"("input string"="写入长度", "regular expression"="0x", "ignore case? (F)"=TRUE) -> ("before match"=w404:string, "after match"=w400:string, "offset past match"=w401:i32)  [unwired: 3 in, 2 out]
            n291 = case shown="-1" w401 {
              tunnel: w400 -> [w648 _]
              tunnel: [w646 w650] -> w388
              tunnel: w404 -> [_ w649]
              frame 0, Default {
                n292 = Hexadecimal String To Number(string=w648, default (0uL)=u8 0 ("default (0 I32)")) -> (number=w646:u8)  [unwired: 1 in, 1 out]
              }
              frame -1 {
                n293 = Decimal String To Number(string=w649, default (0L)=u8 0 ("default (0 U32)")) -> (number=w650:u8)  [unwired: 1 in, 1 out]
              }
            }
            n294 = xnode "Match Regular Expression"("input string"="写入地址（16进制）", "regular expression"="0x", "ignore case? (F)"=TRUE) -> ("before match"=w395:string, "after match"=w399:string, "offset past match"=w398:i32)  [unwired: 3 in, 2 out]
            n295 = case shown="-1" w398 {
              tunnel: w399 -> [w528 _]
              tunnel: [w526 w530] -> w386
              tunnel: w395 -> [_ w529]
              frame 0, Default {
                n296 = Hexadecimal String To Number(string=w528, default (0uL)=u16 0 ("default (0 I32)")) -> (number=w526:u16)  [unwired: 1 in, 1 out]
              }
              frame -1 {
                n297 = Decimal String To Number(string=w529, default (0L)=u16 0 ("default (0 U32)")) -> (number=w530:u16)  [unwired: 1 in, 1 out]
              }
            }
            n298 = xnode "Match Regular Expression"("input string"="写入字符串（16进制）", "regular expression"="0x", "ignore case? (F)"=TRUE) -> ("before match"=w390:string, "after match"=w394:string, "offset past match"=w393:i32)  [unwired: 3 in, 2 out]
            n299 = case shown="-1" w393 {
              tunnel: w394 -> [w409 _]
              tunnel: w390 -> [_ w411]
              tunnel: [w410 w411] -> w385
              frame 0, Default {
                n300 = call "string-hexstring-313.vi"("字符串"=w409) -> ("十六进制整型字符串"=w410:string)  [unwired: 10 in]
              }
              frame -1 {
              }
            }
            n301 = String To Byte Array(string=w385) -> (unsigned byte array=w405:u8[])
            n302 = property on="VISA resource name" class="VISAName"() -> ("Value"=w406:refnum<visa-resource-name>)  [unwired: 2 in, 2 out]
            n303 = property on="COM" class="Bool (strict)"() -> ("Value"=w407:bool)  [unwired: 2 in, 2 out]
            n304 = call "xdata_write.vi"("COM"=w407, "VISA name"=w406, "data"=w405, "wLen"=w388, "wAddr"=w386) -> ("return"=→"写入寄存器":i32)  [unwired: 6 in]
          }
        }
      }
      event "寄存器读取": Value Change {
        n305 = event-data() -> ()  [unwired: 1 in, 6 out]
        n306 = flat-sequence {
          frame #0 {
            n307 = xnode "Match Regular Expression"("input string"="读取地址（16进制）", "regular expression"="0x", "ignore case? (F)"=TRUE) -> ("before match"=w779:string, "after match"=w775:string, "offset past match"=w776:i32)  [unwired: 3 in, 2 out]
            n308 = xnode "Match Regular Expression"("input string"="读取长度", "regular expression"="0x", "ignore case? (F)"=TRUE) -> ("before match"=w770:string, "after match"=w774:string, "offset past match"=w773:i32)  [unwired: 3 in, 2 out]
            n309 = case shown="0, Default" w776 {
              tunnel: w775 -> [w909 _]
              tunnel: [w907 w911] -> w768
              tunnel: w779 -> [_ w910]
              frame 0, Default {
                n310 = Hexadecimal String To Number(string=w909, default (0uL)=u16 0 ("default (0 I32)")) -> (number=w907:u16)  [unwired: 1 in, 1 out]
              }
              frame -1 {
                n311 = Decimal String To Number(string=w910, default (0L)=u16 0 ("default (0 U32)")) -> (number=w911:u16)  [unwired: 1 in, 1 out]
              }
            }
            n312 = case shown="0, Default" w773 {
              tunnel: w774 -> [w789 _]
              tunnel: [w787 w791] -> w766
              tunnel: w770 -> [_ w790]
              frame 0, Default {
                n313 = Hexadecimal String To Number(string=w789, default (0uL)=u8 0 ("default (0 I32)")) -> (number=w787:u8)  [unwired: 1 in, 1 out]
              }
              frame -1 {
                n314 = Decimal String To Number(string=w790, default (0L)=u8 0 ("default (0 U32)")) -> (number=w791:u8)  [unwired: 1 in, 1 out]
              }
            }
            n315 = Initialize Array(u8 0 ("element"), w766) -> (w785:u8[])
            n316 = property on="VISA resource name" class="VISAName"() -> ("Value"=w783:refnum<visa-resource-name>)  [unwired: 2 in, 2 out]
            n317 = property on="COM" class="Bool (strict)"() -> ("Value"=w782:bool)  [unwired: 2 in, 2 out]
            n318 = call "xdata_read.vi"("COM"=w782, "VISA name"=w783, "data"=w785, "wLen"=w766, "wAddr"=w768) -> ("data out"=w780:u8[], "return"=→"读取寄存器":i32)  [unwired: 5 in]
            n319 = Byte Array To String(unsigned byte array=w780) -> (string=→"读取字符串（16进制）":string)
          }
        }
      }
      event "get_vtemp": Value Change {
        n320 = event-data() -> ()  [unwired: 1 in, 6 out]
        n321 = flat-sequence {
          frame #0 {
            n322 = property on="COM" class="Bool (strict)"() -> ("Value"=w1027:bool)  [unwired: 2 in, 2 out]
            n323 = property on="VISA resource name" class="VISAName"() -> ("Value"=w1028:refnum<visa-resource-name>)  [unwired: 2 in, 2 out]
            n324 = call "get_vtemp.vi"("COM"=w1027, "VISA name"=w1028, "cmd_std_header_t"=T3 {"byCmdType"=13, "bySubCmd"=139, "byPara"=0, "byAddr_h"=0, "byAddr_l"=0, "byAddr_ll"=0, "byLen_h"=0, "byLen_l"=0}) -> ("data out"=w1036:u8[], "return"=→"return":i32)  [unwired: 7 in]
            n325 = Index Array(array=w1036, index #1=0 ("index"), index #2=1 ("index")) -> (element #1=w1033:u8, element #2=w1030:u8)
            n326 = Multiply(x=u16 256, y=w1033) -> (x*y=w1031:u16)
            n327 = Add(x=w1031, y=w1030) -> (x+y=→"vtemp":u16)
          }
        }
      }
      event "standard_send": Value Change {
        n328 = event-data() -> ()  [unwired: 1 in, 6 out]
        n329 = flat-sequence {
          frame #0 {
            n330 = local read "Enum"() -> (w1046:enum16{"number", "hex", "string"})
            n331 = xnode "Match Regular Expression"("input string"="std_byCmdType", "regular expression"="0x", "ignore case? (F)"=TRUE) -> ("before match"=w1081:string, "after match"=w1077:string, "offset past match"=w1078:i32)  [unwired: 3 in, 2 out]
            n332 = xnode "Match Regular Expression"("input string"="std_bySubCmd", "regular expression"="0x", "ignore case? (F)"=TRUE) -> ("before match"=w1082:string, "after match"=w1088:string, "offset past match"=w1087:i32)  [unwired: 3 in, 2 out]
            n333 = case shown="\"string\"" w1046 {
              tunnel: ["data_in" w1101 w1105] -> w1044
              frame "number", Default {
              }
              frame "hex" {
                n334 = local read "String_in"() -> (w1102:string)
                n335 = call "string-hexstring-313.vi"("字符串"=w1102) -> ("十六进制整型字符串"=w1103:string)  [unwired: 10 in]
                n336 = String To Byte Array(string=w1103) -> (unsigned byte array=w1101:u8[])
              }
              frame "string" {
                n337 = local read "String_in"() -> (w1104:string)
                n338 = String To Byte Array(string=w1104) -> (unsigned byte array=w1105:u8[])
              }
            }
            n339 = xnode "Match Regular Expression"("input string"="std_byPara", "regular expression"="0x", "ignore case? (F)"=TRUE) -> ("before match"=w1074:string, "after match"=w1070:string, "offset past match"=w1071:i32)  [unwired: 3 in, 2 out]
            n340 = case shown="-1" w1078 {
              tunnel: w1077 -> [w1588 _]
              tunnel: [w1586 w1590] -> w1076
              tunnel: w1081 -> [_ w1589]
              frame 0, Default {
                n341 = Hexadecimal String To Number(string=w1588, default (0uL)=u8 0 ("default (0 I32)")) -> (number=w1586:u8)  [unwired: 1 in, 1 out]
              }
              frame -1 {
                n342 = Decimal String To Number(string=w1589, default (0L)=u8 0 ("default (0 U32)")) -> (number=w1590:u8)  [unwired: 1 in, 1 out]
              }
            }
            n343 = xnode "Match Regular Expression"("input string"="std_byAddr_h", "regular expression"="0x", "ignore case? (F)"=TRUE) -> ("before match"=w1063:string, "after match"=w1067:string, "offset past match"=w1066:i32)  [unwired: 3 in, 2 out]
            n344 = xnode "Match Regular Expression"("input string"="std_wAddr", "regular expression"="0x", "ignore case? (F)"=TRUE) -> ("before match"=w1060:string, "after match"=w1056:string, "offset past match"=w1057:i32)  [unwired: 3 in, 2 out]
            n345 = case shown="-1" w1087 {
              tunnel: w1088 -> [w1708 _]
              tunnel: [w1706 w1710] -> w1083
              tunnel: w1082 -> [_ w1709]
              frame 0, Default {
                n346 = Hexadecimal String To Number(string=w1708, default (0uL)=u8 0 ("default (0 I32)")) -> (number=w1706:u8)  [unwired: 1 in, 1 out]
              }
              frame -1 {
                n347 = Decimal String To Number(string=w1709, default (0L)=u8 0 ("default (0 U32)")) -> (number=w1710:u8)  [unwired: 1 in, 1 out]
              }
            }
            n348 = case shown="-1" w1071 {
              tunnel: w1070 -> [w1468 _]
              tunnel: [w1466 w1470] -> w1068
              tunnel: w1074 -> [_ w1469]
              frame 0, Default {
                n349 = Hexadecimal String To Number(string=w1468, default (0uL)=u8 0 ("default (0 I32)")) -> (number=w1466:u8)  [unwired: 1 in, 1 out]
              }
              frame -1 {
                n350 = Decimal String To Number(string=w1469, default (0L)=u8 0 ("default (0 U32)")) -> (number=w1470:u8)  [unwired: 1 in, 1 out]
              }
            }
            n351 = xnode "Match Regular Expression"("input string"="std_wLength", "regular expression"="0x", "ignore case? (F)"=TRUE) -> ("before match"=w1049:string, "after match"=w1053:string, "offset past match"=w1052:i32)  [unwired: 3 in, 2 out]
            n352 = case shown="0, Default" w1066 {
              tunnel: w1067 -> [w1348 _]
              tunnel: [w1346 w1350] -> w1061
              tunnel: w1063 -> [_ w1349]
              frame 0, Default {
                n353 = Hexadecimal String To Number(string=w1348, default (0uL)=u8 0 ("default (0 I32)")) -> (number=w1346:u8)  [unwired: 1 in, 1 out]
              }
              frame -1 {
                n354 = Decimal String To Number(string=w1349, default (0L)=u8 0 ("default (0 U32)")) -> (number=w1350:u8)  [unwired: 1 in, 1 out]
              }
            }
            n355 = case shown="-1" w1057 {
              tunnel: w1056 -> [w1228 _]
              tunnel: [w1226 w1230] -> w1055
              tunnel: w1060 -> [_ w1229]
              frame 0, Default {
                n356 = Hexadecimal String To Number(string=w1228, default (0uL)=u16 0 ("default (0 I32)")) -> (number=w1226:u16)  [unwired: 1 in, 1 out]
              }
              frame -1 {
                n357 = Decimal String To Number(string=w1229, default (0L)=u16 0 ("default (0 U32)")) -> (number=w1230:u16)  [unwired: 1 in, 1 out]
              }
            }
            n358 = case shown="-1" w1052 {
              tunnel: w1053 -> [w1108 _]
              tunnel: [w1106 w1110] -> w1047
              tunnel: w1049 -> [_ w1109]
              frame 0, Default {
                n359 = Hexadecimal String To Number(string=w1108, default (0uL)=u16 0 ("default (0 I32)")) -> (number=w1106:u16)  [unwired: 1 in, 1 out]
              }
              frame -1 {
                n360 = Decimal String To Number(string=w1109, default (0L)=u16 0 ("default (0 U32)")) -> (number=w1110:u16)  [unwired: 1 in, 1 out]
              }
            }
            n361 = Split Number(x=w1055) -> (hi(x)=w1042:u8, lo(x)=w1041:u8)
            n362 = Split Number(x=w1047) -> (hi(x)=w1040:u8, lo(x)=w1039:u8)
            n363 = Join Numbers(hi=w1042, lo=w1041) -> ((hi.lo)=w1090:u16)
            n364 = Join Numbers(hi=w1068, lo=w1061) -> ((hi.lo)=w1093:u16)
            n365 = Bundle By Name(cluster="cmd_std_header_t", "byCmdType"=w1076, "bySubCmd"=w1083, "byPara"=w1068, "byAddr_h"=w1061, "byAddr_l"=w1042, "byAddr_ll"=w1041, "byLen_h"=w1040, "byLen_l"=w1039) -> (w1094:T3)
            n366 = property on="VISA resource name" class="VISAName"() -> ("Value"=w1097:refnum<visa-resource-name>)  [unwired: 2 in, 2 out]
            n367 = property on="COM" class="Bool (strict)"() -> ("Value"=w1096:bool)  [unwired: 2 in, 2 out]
            n368 = Join Numbers(hi=w1093, lo=w1090) -> ((hi.lo)=w1092:u32)
            n369 = Join Numbers(hi=w1040, lo=w1039) -> ((hi.lo)=w1089:u16)
            n370 = case shown="False" "Boolean" {
              tunnel: [w1098 "new_dead_pix"] -> w1043
              tunnel: w1044 -> [w1098 _]
              frame False {
              }
              frame True {
              }
            }
            n371 = call "standard_cmd_write.vi"("COM"=w1096, "VISA name"=w1097, "data"=w1043, "dwLen"=w1089, "dwAddr"=w1092, "cmd_std_header_t"=w1094) -> ("return"=→"standard_send_return":i32)  [unwired: 5 in]
          }
        }
      }
      event "加载到data_in": Value Change {
        n372 = event-data() -> ()  [unwired: 1 in, 6 out]
        n373 = flat-sequence {
          frame #0 {
            n374 = Initialize Array("数值", "长度") -> (w1826:u8[])
            n375 = property on="data_in" class="Arr (strict)"("Value"=w1826) -> ()  [unwired: 2 in, 2 out]
          }
        }
      }
      event "standard_get": Value Change {
        n376 = event-data() -> ()  [unwired: 1 in, 6 out]
        n377 = flat-sequence {
          frame #0 {
            w1829 = u8 0 ("byLen_l")
            n378 = property on="std_wAddr" class="Str"() -> ("Value"=w1835:string)  [unwired: 2 in, 2 out]
            n379 = property on="std_wLength" class="Str"() -> ("Value"=w1845:string)  [unwired: 2 in, 2 out]
            n380 = property on="std_bySubCmd" class="Str"() -> ("Value"=w1841:string)  [unwired: 2 in, 2 out]
            n381 = property on="std_byPara" class="Str"() -> ("Value"=w1839:string)  [unwired: 2 in, 2 out]
            n382 = property on="std_byAddr_h" class="Str"() -> ("Value"=w1837:string)  [unwired: 2 in, 2 out]
            n383 = property on="std_byCmdType" class="Str"() -> ("Value"=w1843:string)  [unwired: 2 in, 2 out]
            n384 = xnode "Match Regular Expression"("input string"=w1843, "regular expression"="0x", "ignore case? (F)"=TRUE) -> ("before match"=w1870:string, "after match"=w1866:string, "offset past match"=w1867:i32)  [unwired: 3 in, 2 out]
            n385 = xnode "Match Regular Expression"("input string"=w1841, "regular expression"="0x", "ignore case? (F)"=TRUE) -> ("before match"=w1871:string, "after match"=w1875:string, "offset past match"=w1874:i32)  [unwired: 3 in, 2 out]
            n386 = xnode "Match Regular Expression"("input string"=w1839, "regular expression"="0x", "ignore case? (F)"=TRUE) -> ("before match"=w1865:string, "after match"=w1861:string, "offset past match"=w1862:i32)  [unwired: 3 in, 2 out]
            n387 = case shown="-1" w1867 {
              tunnel: w1866 -> [w2378 _]
              tunnel: [w2376 w2380] -> w1842
              tunnel: w1870 -> [_ w2379]
              frame 0, Default {
                n388 = Hexadecimal String To Number(string=w2378, default (0uL)=u8 0 ("default (0 I32)")) -> (number=w2376:u8)  [unwired: 1 in, 1 out]
              }
              frame -1 {
                n389 = Decimal String To Number(string=w2379, default (0L)=u8 0 ("default (0 U32)")) -> (number=w2380:u8)  [unwired: 1 in, 1 out]
              }
            }
            n390 = xnode "Match Regular Expression"("input string"=w1837, "regular expression"="0x", "ignore case? (F)"=TRUE) -> ("before match"=w1856:string, "after match"=w1860:string, "offset past match"=w1859:i32)  [unwired: 3 in, 2 out]
            n391 = xnode "Match Regular Expression"("input string"=w1835, "regular expression"="0x", "ignore case? (F)"=TRUE) -> ("before match"=w1855:string, "after match"=w1851:string, "offset past match"=w1852:i32)  [unwired: 3 in, 2 out]
            n392 = case shown="-1" w1874 {
              tunnel: w1875 -> [w2498 _]
              tunnel: [w2496 w2500] -> w1840
              tunnel: w1871 -> [_ w2499]
              frame 0, Default {
                n393 = Hexadecimal String To Number(string=w2498, default (0uL)=u8 0 ("default (0 I32)")) -> (number=w2496:u8)  [unwired: 1 in, 1 out]
              }
              frame -1 {
                n394 = Decimal String To Number(string=w2499, default (0L)=u8 0 ("default (0 U32)")) -> (number=w2500:u8)  [unwired: 1 in, 1 out]
              }
            }
            n395 = case shown="-1" w1862 {
              tunnel: w1861 -> [w2258 _]
              tunnel: [w2256 w2260] -> w1838
              tunnel: w1865 -> [_ w2259]
              frame 0, Default {
                n396 = Hexadecimal String To Number(string=w2258, default (0uL)=u8 0 ("default (0 I32)")) -> (number=w2256:u8)  [unwired: 1 in, 1 out]
              }
              frame -1 {
                n397 = Decimal String To Number(string=w2259, default (0L)=u8 0 ("default (0 U32)")) -> (number=w2260:u8)  [unwired: 1 in, 1 out]
              }
            }
            n398 = xnode "Match Regular Expression"("input string"=w1845, "regular expression"="0x", "ignore case? (F)"=TRUE) -> ("before match"=w1846:string, "after match"=w1850:string, "offset past match"=w1849:i32)  [unwired: 3 in, 2 out]
            n399 = case shown="0, Default" w1859 {
              tunnel: w1860 -> [w2138 _]
              tunnel: [w2136 w2140] -> w1836
              tunnel: w1856 -> [_ w2139]
              frame 0, Default {
                n400 = Hexadecimal String To Number(string=w2138, default (0uL)=u8 0 ("default (0 I32)")) -> (number=w2136:u8)  [unwired: 1 in, 1 out]
              }
              frame -1 {
                n401 = Decimal String To Number(string=w2139, default (0L)=u8 0 ("default (0 U32)")) -> (number=w2140:u8)  [unwired: 1 in, 1 out]
              }
            }
            n402 = case shown="-1" w1852 {
              tunnel: w1851 -> [w2018 _]
              tunnel: [w2016 w2020] -> w1832
              tunnel: w1855 -> [_ w2019]
              frame 0, Default {
                n403 = Hexadecimal String To Number(string=w2018, default (0uL)=u16 0 ("default (0 I32)")) -> (number=w2016:u16)  [unwired: 1 in, 1 out]
              }
              frame -1 {
                n404 = Decimal String To Number(string=w2019, default (0L)=u16 0 ("default (0 U32)")) -> (number=w2020:u16)  [unwired: 1 in, 1 out]
              }
            }
            n405 = case shown="-1" w1849 {
              tunnel: w1850 -> [w1898 _]
              tunnel: [w1896 w1900] -> w1844
              tunnel: w1846 -> [_ w1899]
              frame 0, Default {
                n406 = Hexadecimal String To Number(string=w1898, default (0uL)=u16 0 ("default (0 I32)")) -> (number=w1896:u16)  [unwired: 1 in, 1 out]
              }
              frame -1 {
                n407 = Decimal String To Number(string=w1899, default (0L)=u16 0 ("default (0 U32)")) -> (number=w1900:u16)  [unwired: 1 in, 1 out]
              }
            }
            n408 = property on="cmd_std_header_t" class="Clust (strict)"() -> ("Value"=w1883:T3)  [unwired: 2 in, 2 out]
            n409 = Split Number(x=w1832) -> (hi(x)=w1831:u8, lo(x)=w1830:u8)
            n410 = Join Numbers(hi=w1838, lo=w1836) -> ((hi.lo)=w1884:u16)
            n411 = property on="VISA resource name" class="VISAName"() -> ("Value"=w1881:refnum<visa-resource-name>)  [unwired: 2 in, 2 out]
            n412 = property on="COM" class="Bool (strict)"() -> ("Value"=w1880:bool)  [unwired: 2 in, 2 out]
            n413 = Join Numbers(hi=w1884, lo=w1832) -> ((hi.lo)=w1879:u32)
            n414 = local read "Enum"() -> (w1834:enum16{"number", "hex", "string"})
            n415 = Bundle By Name(cluster=w1883, "byCmdType"=w1842, "bySubCmd"=w1840, "byPara"=w1838, "byAddr_h"=w1836, "byAddr_l"=w1831, "byAddr_ll"=w1830, "byLen_h"=w1829, "byLen_l"=w1829) -> (w1882:T3)
            n416 = Initialize Array(u8 0 ("element"), w1844) -> (w1876:u8[])
            n417 = call "standard_cmd_read.vi"("COM"=w1880, "VISA name"=w1881, "data"=w1876, "dwLen"=w1844, "dwAddr"=w1879, "cmd_std_header_t"=w1882) -> ("return"=→"standard_get_return":i32, "data out"=w1833:u8[])  [unwired: 4 in]
            n418 = case shown="\"hex\"" w1834 {
              tunnel: w1833 -> [w1885 w1888 w1894]
              frame "number", Default {
                "data_out" <- w1885
              }
              frame "hex" {
                n419 = for {
                  tunnel: w1888 -> [w1893] mode=indexing
                  shift-right: [w1892] -> w1886
                  shift-left: "" -> [w1891]
                  n420 = Number To Hexadecimal String(1:i16 2 ("width (-)"), 2:w1893) -> (0:w1890:string)
                  n421 = Concatenate Strings(w1891, w1890) -> (w1892:string)
                }
                n422 = local write "String_out"(w1886) -> ()
              }
              frame "string" {
                n423 = Byte Array To String(unsigned byte array=w1894) -> (string=w1895:string)
                n424 = local write "String_out"(w1895) -> ()
              }
            }
          }
        }
      }
      event "long_send": Value Change {
        n425 = event-data() -> ()  [unwired: 1 in, 6 out]
        n426 = flat-sequence {
          frame #0 {
            n427 = property on="long_byCmd" class="Str"() -> ("Value"=w2618:string)  [unwired: 2 in, 2 out]
            n428 = property on="long_bySubCmd" class="Str"() -> ("Value"=w2619:string)  [unwired: 2 in, 2 out]
            n429 = property on="long_wPara" class="Str"() -> ("Value"=w2620:string)  [unwired: 2 in, 2 out]
            n430 = property on="long_dwAddr1" class="Str"() -> ("Value"=w2625:string)  [unwired: 2 in, 2 out]
            n431 = property on="long_dwAddr2" class="Str"() -> ("Value"=w2627:string)  [unwired: 2 in, 2 out]
            n432 = property on="long_dwLen" class="Str"() -> ("Value"=w2629:string)  [unwired: 2 in, 2 out]
            n433 = xnode "Match Regular Expression"("input string"=w2627, "regular expression"="0x", "ignore case? (F)"=TRUE) -> ("before match"=w2639:string, "after match"=w2635:string, "offset past match"=w2636:i32)  [unwired: 3 in, 2 out]
            n434 = xnode "Match Regular Expression"("input string"=w2629, "regular expression"="0x", "ignore case? (F)"=TRUE) -> ("before match"=w2630:string, "after match"=w2634:string, "offset past match"=w2633:i32)  [unwired: 3 in, 2 out]
            n435 = xnode "Match Regular Expression"("input string"=w2625, "regular expression"="0x", "ignore case? (F)"=TRUE) -> ("before match"=w2640:string, "after match"=w2644:string, "offset past match"=w2643:i32)  [unwired: 3 in, 2 out]
            n436 = xnode "Match Regular Expression"("input string"=w2618, "regular expression"="0x", "ignore case? (F)"=TRUE) -> ("before match"=w2654:string, "after match"=w2650:string, "offset past match"=w2651:i32)  [unwired: 3 in, 2 out]
            n437 = xnode "Match Regular Expression"("input string"=w2619, "regular expression"="0x", "ignore case? (F)"=TRUE) -> ("before match"=w2655:string, "after match"=w2659:string, "offset past match"=w2658:i32)  [unwired: 3 in, 2 out]
            n438 = xnode "Match Regular Expression"("input string"=w2620, "regular expression"="0x", "ignore case? (F)"=TRUE) -> ("before match"=w2649:string, "after match"=w2645:string, "offset past match"=w2646:i32)  [unwired: 3 in, 2 out]
            n439 = case shown="0, Default" w2636 {
              tunnel: w2635 -> [w2799 _]
              tunnel: [w2797 w2801] -> w2626
              tunnel: w2639 -> [_ w2800]
              frame 0, Default {
                n440 = Hexadecimal String To Number(string=w2799, default (0uL)=u32 0 ("default (0 I32)")) -> (number=w2797:u32)  [unwired: 1 in, 1 out]
              }
              frame -1 {
                n441 = Decimal String To Number(string=w2800, default (0L)=u32 0 ("default (0 U32)")) -> (number=w2801:u32)  [unwired: 1 in, 1 out]
              }
            }
            n442 = case shown="0, Default" w2633 {
              tunnel: w2634 -> [w2679 _]
              tunnel: [w2677 w2681] -> w2628
              tunnel: w2630 -> [_ w2680]
              frame 0, Default {
                n443 = Hexadecimal String To Number(string=w2679, default (0uL)=u32 0 ("default (0 I32)")) -> (number=w2677:u32)  [unwired: 1 in, 1 out]
              }
              frame -1 {
                n444 = Decimal String To Number(string=w2680, default (0L)=u32 0 ("default (0 U32)")) -> (number=w2681:u32)  [unwired: 1 in, 1 out]
              }
            }
            n445 = case shown="-1" w2643 {
              tunnel: w2644 -> [w2919 _]
              tunnel: [w2917 w2921] -> w2624
              tunnel: w2640 -> [_ w2920]
              frame 0, Default {
                n446 = Hexadecimal String To Number(string=w2919, default (0uL)=u32 0 ("default (0 I32)")) -> (number=w2917:u32)  [unwired: 1 in, 1 out]
              }
              frame -1 {
                n447 = Decimal String To Number(string=w2920, default (0L)=u32 0 ("default (0 U32)")) -> (number=w2921:u32)  [unwired: 1 in, 1 out]
              }
            }
            n448 = case shown="-1" w2651 {
              tunnel: w2650 -> [w3159 _]
              tunnel: [w3157 w3161] -> w2617
              tunnel: w2654 -> [_ w3160]
              frame 0, Default {
                n449 = Hexadecimal String To Number(string=w3159, default (0uL)=u8 0 ("default (0 I32)")) -> (number=w3157:u8)  [unwired: 1 in, 1 out]
              }
              frame -1 {
                n450 = Decimal String To Number(string=w3160, default (0L)=u8 0 ("default (0 U32)")) -> (number=w3161:u8)  [unwired: 1 in, 1 out]
              }
            }
            n451 = case shown="-1" w2658 {
              tunnel: w2659 -> [w3279 _]
              tunnel: [w3277 w3281] -> w2616
              tunnel: w2655 -> [_ w3280]
              frame 0, Default {
                n452 = Hexadecimal String To Number(string=w3279, default (0uL)=u8 0 ("default (0 I32)")) -> (number=w3277:u8)  [unwired: 1 in, 1 out]
              }
              frame -1 {
                n453 = Decimal String To Number(string=w3280, default (0L)=u8 0 ("default (0 U32)")) -> (number=w3281:u8)  [unwired: 1 in, 1 out]
              }
            }
            n454 = case shown="0, Default" w2646 {
              tunnel: w2645 -> [w3039 _]
              tunnel: [w3037 w3041] -> w2623
              tunnel: w2649 -> [_ w3040]
              frame 0, Default {
                n455 = Hexadecimal String To Number(string=w3039, default (0uL)=u16 0 ("default (0 I32)")) -> (number=w3037:u16)  [unwired: 1 in, 1 out]
              }
              frame -1 {
                n456 = Decimal String To Number(string=w3040, default (0L)=u16 0 ("default (0 U32)")) -> (number=w3041:u16)  [unwired: 1 in, 1 out]
              }
            }
            n457 = Split Number(x=w2623) -> (hi(x)=w2622:u8, lo(x)=w2621:u8)
            n458 = Unbundle By Name("vd_cmd_long_header_t") -> ("byAddr1_hh"=w2664:u8, "byAddr1_h"=w2665:u8, "byAddr1_l"=w2666:u8, "byAddr1_ll"=w2667:u8, "byAddr2_hh"=w2668:u8, "byAddr2_h"=w2669:u8, "byAddr2_l"=w2670:u8, "byAddr2_ll"=w2671:u8, "byLen_hh"=w2672:u8, "byLen_h"=w2673:u8, "byLen_l"=w2674:u8, "byLen_ll"=w2675:u8)
            n459 = Bundle By Name(cluster="vd_cmd_long_header_t", "byCmd"=w2617, "bySubCmd"=w2616, "byParam_h"=w2622, "byParam_l"=w2621, "byAddr1_hh"=w2664, "byAddr1_h"=w2665, "byAddr1_l"=w2666, "byAddr1_ll"=w2667, "byAddr2_hh"=w2668, "byAddr2_h"=w2669, "byAddr2_l"=w2670, "byAddr2_ll"=w2671, "byLen_hh"=w2672, "byLen_h"=w2673, "byLen_l"=w2674, "byLen_ll"=w2675) -> (w2663:T4)
            n460 = property on="VISA resource name" class="VISAName"() -> ("Value"=w2662:refnum<visa-resource-name>)  [unwired: 2 in, 2 out]
            n461 = property on="COM" class="Bool (strict)"() -> ("Value"=w2661:bool)  [unwired: 2 in, 2 out]
            n462 = call "long_cmd_write.vi"("COM"=w2661, "dwLen"=w2628, "VISA name"=w2662, "dwAddr2"=w2626, "dwAddr1"=w2624, "vd_cmd_long_header_t"=w2663) -> ("return"=→"long_send_return":i32)  [unwired: 4 in, 1 out]
          }
        }
      }
      event "long_get": Value Change {
        n463 = event-data() -> ()  [unwired: 1 in, 6 out]
        n464 = flat-sequence {
          frame #0 {
            n465 = xnode "Match Regular Expression"("input string"="long_dwAddr2", "regular expression"="0x", "ignore case? (F)"=TRUE) -> ("before match"=w3420:string, "after match"=w3416:string, "offset past match"=w3417:i32)  [unwired: 3 in, 2 out]
            n466 = xnode "Match Regular Expression"("input string"="long_dwLen", "regular expression"="0x", "ignore case? (F)"=TRUE) -> ("before match"=w3411:string, "after match"=w3415:string, "offset past match"=w3414:i32)  [unwired: 3 in, 2 out]
            n467 = xnode "Match Regular Expression"("input string"="long_dwAddr1", "regular expression"="0x", "ignore case? (F)"=TRUE) -> ("before match"=w3421:string, "after match"=w3425:string, "offset past match"=w3424:i32)  [unwired: 3 in, 2 out]
            n468 = xnode "Match Regular Expression"("input string"="long_byCmd", "regular expression"="0x", "ignore case? (F)"=TRUE) -> ("before match"=w3435:string, "after match"=w3431:string, "offset past match"=w3432:i32)  [unwired: 3 in, 2 out]
            n469 = xnode "Match Regular Expression"("input string"="long_bySubCmd", "regular expression"="0x", "ignore case? (F)"=TRUE) -> ("before match"=w3436:string, "after match"=w3440:string, "offset past match"=w3439:i32)  [unwired: 3 in, 2 out]
            n470 = xnode "Match Regular Expression"("input string"="long_wPara", "regular expression"="0x", "ignore case? (F)"=TRUE) -> ("before match"=w3430:string, "after match"=w3426:string, "offset past match"=w3427:i32)  [unwired: 3 in, 2 out]
            n471 = case shown="0, Default" w3417 {
              tunnel: w3416 -> [w3583 _]
              tunnel: [w3581 w3585] -> w3398
              tunnel: w3420 -> [_ w3584]
              frame 0, Default {
                n472 = Hexadecimal String To Number(string=w3583, default (0uL)=u32 0 ("default (0 I32)")) -> (number=w3581:u32)  [unwired: 1 in, 1 out]
              }
              frame -1 {
                n473 = Decimal String To Number(string=w3584, default (0L)=u32 0 ("default (0 U32)")) -> (number=w3585:u32)  [unwired: 1 in, 1 out]
              }
            }
            n474 = case shown="0, Default" w3414 {
              tunnel: w3415 -> [w3463 _]
              tunnel: [w3461 w3465] -> w3399
              tunnel: w3411 -> [_ w3464]
              frame 0, Default {
                n475 = Hexadecimal String To Number(string=w3463, default (0uL)=u32 0 ("default (0 I32)")) -> (number=w3461:u32)  [unwired: 1 in, 1 out]
              }
              frame -1 {
                n476 = Decimal String To Number(string=w3464, default (0L)=u32 0 ("default (0 U32)")) -> (number=w3465:u32)  [unwired: 1 in, 1 out]
              }
            }
            n477 = case shown="-1" w3424 {
              tunnel: w3425 -> [w3703 _]
              tunnel: [w3701 w3705] -> w3397
              tunnel: w3421 -> [_ w3704]
              frame 0, Default {
                n478 = Hexadecimal String To Number(string=w3703, default (0uL)=u32 0 ("default (0 I32)")) -> (number=w3701:u32)  [unwired: 1 in, 1 out]
              }
              frame -1 {
                n479 = Decimal String To Number(string=w3704, default (0L)=u32 0 ("default (0 U32)")) -> (number=w3705:u32)  [unwired: 1 in, 1 out]
              }
            }
            n480 = case shown="-1" w3432 {
              tunnel: w3431 -> [w3943 _]
              tunnel: [w3941 w3945] -> w3406
              tunnel: w3435 -> [_ w3944]
              frame 0, Default {
                n481 = Hexadecimal String To Number(string=w3943, default (0uL)=u8 0 ("default (0 I32)")) -> (number=w3941:u8)  [unwired: 1 in, 1 out]
              }
              frame -1 {
                n482 = Decimal String To Number(string=w3944, default (0L)=u8 0 ("default (0 U32)")) -> (number=w3945:u8)  [unwired: 1 in, 1 out]
              }
            }
            n483 = case shown="-1" w3439 {
              tunnel: w3440 -> [w4063 _]
              tunnel: [w4061 w4065] -> w3404
              tunnel: w3436 -> [_ w4064]
              frame 0, Default {
                n484 = Hexadecimal String To Number(string=w4063, default (0uL)=u8 0 ("default (0 I32)")) -> (number=w4061:u8)  [unwired: 1 in, 1 out]
              }
              frame -1 {
                n485 = Decimal String To Number(string=w4064, default (0L)=u8 0 ("default (0 U32)")) -> (number=w4065:u8)  [unwired: 1 in, 1 out]
              }
            }
            n486 = case shown="0, Default" w3427 {
              tunnel: w3426 -> [w3823 _]
              tunnel: [w3821 w3825] -> w3403
              tunnel: w3430 -> [_ w3824]
              frame 0, Default {
                n487 = Hexadecimal String To Number(string=w3823, default (0uL)=u16 0 ("default (0 I32)")) -> (number=w3821:u16)  [unwired: 1 in, 1 out]
              }
              frame -1 {
                n488 = Decimal String To Number(string=w3824, default (0L)=u16 0 ("default (0 U32)")) -> (number=w3825:u16)  [unwired: 1 in, 1 out]
              }
            }
            n489 = property on="vd_cmd_long_header_t" class="Clust (strict)"() -> ("Value"=w3460:T4)  [unwired: 2 in, 2 out]
            n490 = Split Number(x=w3403) -> (hi(x)=w3410:u8, lo(x)=w3409:u8)
            n491 = Unbundle By Name(w3460) -> ("byAddr1_hh"=w3448:u8, "byAddr1_h"=w3449:u8, "byAddr1_l"=w3450:u8, "byAddr1_ll"=w3451:u8, "byAddr2_hh"=w3452:u8, "byAddr2_h"=w3453:u8, "byAddr2_l"=w3454:u8, "byAddr2_ll"=w3455:u8, "byLen_hh"=w3456:u8, "byLen_h"=w3457:u8, "byLen_l"=w3458:u8, "byLen_ll"=w3459:u8)
            n492 = Initialize Array(u8 0 ("element"), w3399) -> (w3443:u8[])
            n493 = Bundle By Name(cluster=w3460, "byCmd"=w3406, "bySubCmd"=w3404, "byParam_h"=w3410, "byParam_l"=w3409, "byAddr1_hh"=w3448, "byAddr1_h"=w3449, "byAddr1_l"=w3450, "byAddr1_ll"=w3451, "byAddr2_hh"=w3452, "byAddr2_h"=w3453, "byAddr2_l"=w3454, "byAddr2_ll"=w3455, "byLen_hh"=w3456, "byLen_h"=w3457, "byLen_l"=w3458, "byLen_ll"=w3459) -> (w3447:T4)
            n494 = property on="VISA resource name" class="VISAName"() -> ("Value"=w3446:refnum<visa-resource-name>)  [unwired: 2 in, 2 out]
            n495 = property on="COM" class="Bool (strict)"() -> ("Value"=w3445:bool)  [unwired: 2 in, 2 out]
            n496 = call "long_cmd_read.vi"("data"=w3443, "COM"=w3445, "dwLen"=w3399, "VISA name"=w3446, "dwAddr2"=w3398, "dwAddr1"=w3397, "vd_cmd_long_header_t"=w3447) -> ("data out"=→"long_data out":u8[], "return"=→"long_get_return":i32)  [unwired: 2 in, 1 out]
          }
        }
      }
      event "osd_send": Value Change {
        n497 = event-data() -> ()  [unwired: 1 in, 6 out]
        n498 = flat-sequence {
          frame #0 {
            n499 = xnode "Match Regular Expression"("input string"="osd_byPara", "regular expression"="0x", "ignore case? (F)"=TRUE) -> ("before match"=w4189:string, "after match"=w4193:string, "offset past match"=w4192:i32)  [unwired: 3 in, 2 out]
            n500 = xnode "Match Regular Expression"("input string"="osd_byCmd", "regular expression"="0x", "ignore case? (F)"=TRUE) -> ("before match"=w4203:string, "after match"=w4199:string, "offset past match"=w4200:i32)  [unwired: 3 in, 2 out]
            n501 = xnode "Match Regular Expression"("input string"="osd_bySubcmd", "regular expression"="0x", "ignore case? (F)"=TRUE) -> ("before match"=w4204:string, "after match"=w4208:string, "offset past match"=w4207:i32)  [unwired: 3 in, 2 out]
            n502 = xnode "Match Regular Expression"("input string"="osd_byIndex", "regular expression"="0x", "ignore case? (F)"=TRUE) -> ("before match"=w4198:string, "after match"=w4194:string, "offset past match"=w4195:i32)  [unwired: 3 in, 2 out]
            n503 = case shown="0, Default" w4192 {
              tunnel: w4193 -> [w4215 _]
              tunnel: [w4213 w4217] -> w4184
              tunnel: w4189 -> [_ w4216]
              frame 0, Default {
                n504 = Hexadecimal String To Number(string=w4215, default (0uL)=u8 0 ("default (0 I32)")) -> (number=w4213:u8)  [unwired: 1 in, 1 out]
              }
              frame -1 {
                n505 = Decimal String To Number(string=w4216, default (0L)=u8 0 ("default (0 U32)")) -> (number=w4217:u8)  [unwired: 1 in, 1 out]
              }
            }
            n506 = case shown="-1" w4200 {
              tunnel: w4199 -> [w4455 _]
              tunnel: [w4453 w4457] -> w4182
              tunnel: w4203 -> [_ w4456]
              frame 0, Default {
                n507 = Hexadecimal String To Number(string=w4455, default (0uL)=u8 0 ("default (0 I32)")) -> (number=w4453:u8)  [unwired: 1 in, 1 out]
              }
              frame -1 {
                n508 = Decimal String To Number(string=w4456, default (0L)=u8 0 ("default (0 U32)")) -> (number=w4457:u8)  [unwired: 1 in, 1 out]
              }
            }
            n509 = case shown="-1" w4207 {
              tunnel: w4208 -> [w4575 _]
              tunnel: [w4573 w4577] -> w4181
              tunnel: w4204 -> [_ w4576]
              frame 0, Default {
                n510 = Hexadecimal String To Number(string=w4575, default (0uL)=u8 0 ("default (0 I32)")) -> (number=w4573:u8)  [unwired: 1 in, 1 out]
              }
              frame -1 {
                n511 = Decimal String To Number(string=w4576, default (0L)=u8 0 ("default (0 U32)")) -> (number=w4577:u8)  [unwired: 1 in, 1 out]
              }
            }
            n512 = case shown="-1" w4195 {
              tunnel: w4194 -> [w4335 _]
              tunnel: [w4333 w4337] -> w4183
              tunnel: w4198 -> [_ w4336]
              frame 0, Default {
                n513 = Hexadecimal String To Number(string=w4335, default (0uL)=u8 0 ("default (0 I32)")) -> (number=w4333:u8)  [unwired: 1 in, 1 out]
              }
              frame -1 {
                n514 = Decimal String To Number(string=w4336, default (0L)=u8 0 ("default (0 U32)")) -> (number=w4337:u8)  [unwired: 1 in, 1 out]
              }
            }
            n515 = property on="VISA resource name" class="VISAName"() -> ("Value"=w4211:refnum<visa-resource-name>)  [unwired: 2 in, 2 out]
            n516 = property on="COM" class="Bool (strict)"() -> ("Value"=w4210:bool)  [unwired: 2 in, 2 out]
            n517 = call "osd_send_data.vi"("COM"=w4210, "bypara"=w4184, "VISA name"=w4211, "byIndex"=w4183, "pbyData"="osd_data_in", "bySubcmd"=w4181, "byCmd"=w4182) -> ("return"=→"osd_send_return":i32)  [unwired: 4 in]
          }
        }
      }
      event "osd_get": Value Change {
        n518 = event-data() -> ()  [unwired: 1 in, 6 out]
        n519 = flat-sequence {
          frame #0 {
            n520 = property on="osd_byCmd" class="Str"() -> ("Value"=w4700:string)  [unwired: 2 in, 2 out]
            n521 = property on="osd_byPara" class="Str"() -> ("Value"=w4697:string)  [unwired: 2 in, 2 out]
            n522 = property on="osd_bySubcmd" class="Str"() -> ("Value"=w4699:string)  [unwired: 2 in, 2 out]
            n523 = property on="osd_byIndex" class="Str"() -> ("Value"=w4698:string)  [unwired: 2 in, 2 out]
            n524 = xnode "Match Regular Expression"("input string"=w4697, "regular expression"="0x", "ignore case? (F)"=TRUE) -> ("before match"=w4701:string, "after match"=w4705:string, "offset past match"=w4704:i32)  [unwired: 3 in, 2 out]
            n525 = xnode "Match Regular Expression"("input string"=w4700, "regular expression"="0x", "ignore case? (F)"=TRUE) -> ("before match"=w4715:string, "after match"=w4711:string, "offset past match"=w4712:i32)  [unwired: 3 in, 2 out]
            n526 = xnode "Match Regular Expression"("input string"=w4699, "regular expression"="0x", "ignore case? (F)"=TRUE) -> ("before match"=w4716:string, "after match"=w4720:string, "offset past match"=w4719:i32)  [unwired: 3 in, 2 out]
            n527 = xnode "Match Regular Expression"("input string"=w4698, "regular expression"="0x", "ignore case? (F)"=TRUE) -> ("before match"=w4710:string, "after match"=w4706:string, "offset past match"=w4707:i32)  [unwired: 3 in, 2 out]
            n528 = case shown="0, Default" w4704 {
              tunnel: w4705 -> [w4727 _]
              tunnel: [w4725 w4729] -> w4693
              tunnel: w4701 -> [_ w4728]
              frame 0, Default {
                n529 = Hexadecimal String To Number(string=w4727, default (0uL)=u8 0 ("default (0 I32)")) -> (number=w4725:u8)  [unwired: 1 in, 1 out]
              }
              frame -1 {
                n530 = Decimal String To Number(string=w4728, default (0L)=u8 0 ("default (0 U32)")) -> (number=w4729:u8)  [unwired: 1 in, 1 out]
              }
            }
            n531 = case shown="-1" w4712 {
              tunnel: w4711 -> [w4967 _]
              tunnel: [w4965 w4969] -> w4696
              tunnel: w4715 -> [_ w4968]
              frame 0, Default {
                n532 = Hexadecimal String To Number(string=w4967, default (0uL)=u8 0 ("default (0 I32)")) -> (number=w4965:u8)  [unwired: 1 in, 1 out]
              }
              frame -1 {
                n533 = Decimal String To Number(string=w4968, default (0L)=u8 0 ("default (0 U32)")) -> (number=w4969:u8)  [unwired: 1 in, 1 out]
              }
            }
            n534 = case shown="-1" w4719 {
              tunnel: w4720 -> [w5087 _]
              tunnel: [w5085 w5089] -> w4695
              tunnel: w4716 -> [_ w5088]
              frame 0, Default {
                n535 = Hexadecimal String To Number(string=w5087, default (0uL)=u8 0 ("default (0 I32)")) -> (number=w5085:u8)  [unwired: 1 in, 1 out]
              }
              frame -1 {
                n536 = Decimal String To Number(string=w5088, default (0L)=u8 0 ("default (0 U32)")) -> (number=w5089:u8)  [unwired: 1 in, 1 out]
              }
            }
            n537 = case shown="-1" w4707 {
              tunnel: w4706 -> [w4847 _]
              tunnel: [w4845 w4849] -> w4694
              tunnel: w4710 -> [_ w4848]
              frame 0, Default {
                n538 = Hexadecimal String To Number(string=w4847, default (0uL)=u8 0 ("default (0 I32)")) -> (number=w4845:u8)  [unwired: 1 in, 1 out]
              }
              frame -1 {
                n539 = Decimal String To Number(string=w4848, default (0L)=u8 0 ("default (0 U32)")) -> (number=w4849:u8)  [unwired: 1 in, 1 out]
              }
            }
            n540 = property on="VISA resource name" class="VISAName"() -> ("Value"=w4724:refnum<visa-resource-name>)  [unwired: 2 in, 2 out]
            n541 = property on="COM" class="Bool (strict)"() -> ("Value"=w4723:bool)  [unwired: 2 in, 2 out]
            n542 = call "osd_get_data.vi"("bypara"=w4693, "COM"=w4723, "byIndex"=w4694, "VISA name"=w4724, "bySubcmd"=w4695, "byCmd"=w4696) -> ("data out"=→"osd_data out":u8[], "return"=→"osd_get_return":i32)  [unwired: 4 in]
          }
        }
      }
      event "data数组清空": Value Change {
        n543 = event-data() -> ()  [unwired: 1 in, 6 out]
        n544 = flat-sequence {
          frame #0 {
            n545 = property on="data_out" class="Arr (strict)"("Value"=u8[] [] ("data_out")) -> ()  [unwired: 2 in, 2 out]
            n546 = property on="long_data out" class="Arr (strict)"("Value"=u8[] [] ("long_data out")) -> ()  [unwired: 2 in, 2 out]
            n547 = property on="data_in" class="Arr (strict)"("Value"=u8[] [] ("data_in")) -> ()  [unwired: 2 in, 2 out]
            n548 = property on="osd_data_in" class="Arr (strict)"("Value"=u8[] [] ("data_in")) -> ()  [unwired: 2 in, 2 out]
          }
        }
      }
    }
  }
